vi "AK Befehl Auswerten_MEXA.vi"(10 "Array":string[](array[string])) -> (2 "String für schreiben":string)   [LabVIEW 2020, in "AK-Schnittstelle.lvlib"]
uses:
  AK-Schnittstelle.lvlib
  Aktionen Stoernummern pruefen.ctl
  Aktionen Zustandsfehlerinformation.ctl
  AK Namen Aktionen.ctl
  Seiten/CalGas Aufschaltung/FGV CalGas Aktionen.ctl
  Seiten/FT-IR/Aktion FGV Rezepte wechseln.ctl
  Seiten/FT-IR/AK-manuell.ctl
  Amium PNS/Aktion FGV Amium Daten.ctl
  Seiten/System Einstellungen V2/Aktioen FGV System Konstanten.ctl
  Aktionen Gespeicherte Werte.ctl
  Seiten/System Einstellungen V2/Aktioen FGV System.ctl
  Funktionstasten/Funktionstasten-Aktion.ctl
  Funktionstasten/Zustaende.ctl
  Schedule Modul/Aktion FGV Scheduler Status.ctl
  Seiten/FT-IR/FGV FT-IR Aktionen.ctl
  Analysator Definition/FGV Analysator Definition Aktionen.ctl
  Seiten/FT-IR/FGV FT-IR Diagnose Aktionen.ctl
  Seiten/Erweiterte Konfig/Status Dichtheitstest Aktionen.ctl
  Seiten/Erweiterte Konfig/FGV PID Aktionen.ctl
  Seiten/Anlagengrenzwerte/FGV Anlagengrenzwerte Aktionen.ctl
  Funktionstasten/Betriebsart.ctl
  Amium PNS/AK Kommunikation/Amium Kommandos verwalten Aktionen.ctl
  Seiten/Log Konfig/Aktionen Trigger.ctl
  Messdaten/Aktionen FGV Messdaten.ctl
  Seiten/FT-IR/TOOLweb Interface Library/TOOLweb Rezept wechseln.vi
  Seiten/Erweiterte Konfig/Dichtheitstest.vi
  Funktionstasten/Funktionstasten.lvlib
  Seiten/Log Konfig/LogKonfig.lvlib
  Seiten/FT-IR/FT-IR.lvlib
  Seiten/FT-IR/FGV FT-IR Gasliste Aktionen.ctl
  Messdaten/Messdaten.lvlib
  Seiten/System Einstellungen V2/System Einstellungen V2.lvlib
  Seiten/Erweiterte Konfig/Erweiterte Konfig.lvlib
  Allgemein/allgemeine Sub-VIs.lvlib
  cRIO/PC/Kommunikation mit cRIO.lvlib
  Seiten/Anlagengrenzwerte/Anlagengrenzwerte.lvlib
  Seiten/FT-IR/TOOLweb Interface Library/TOOLweb Interface.lvlib
  Analysator Definition/Analysator Definition.lvlib
  Amium PNS/AK Kommunikation/AK Kommunikation.lvlib
  Seiten/CalGas Aufschaltung/CalGas Aufschaltung.lvlib
  Amium PNS/Amium PNS.lvlib
  Schedule Modul/Schedule Modul.lvlib
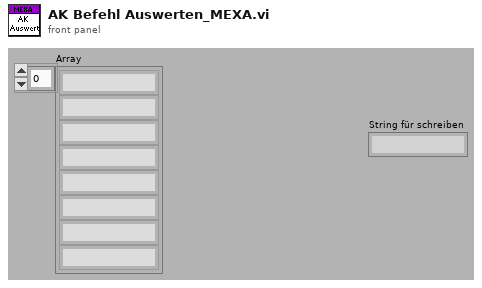
[diagram p1: front panel]
types:
  T1 = typedef "AK-Schnittstelle.lvlib/Aktionen Stoernummern pruefen.ctl" = enum16{"lesen", "prüfen"}
  T2 = typedef "AK-Schnittstelle.lvlib/Aktionen Zustandsfehlerinformation.ctl" = enum16{"OK", "Offline", "Busy", "Syntax Error", "Datenfehler"}
  T3 = typedef "AK-Schnittstelle.lvlib/AK Namen Aktionen.ctl" = enum16{"lesen", "laden", "speichern Namen", "AK Namen", "Liste erstellen", "EKFG erstellen", "speichern EKFG", "EKFG schreiben", "Neuen Eintrag erzeugen"}
  T4 = typedef "CalGas Aufschaltung.lvlib/FGV CalGas Aktionen.ctl" = enum16{"lesen", "Analysator Auswahl", "Def.CalGas", "Aufschaltung CalGas", "laden", "speichern", "KAL extrahieren"}
  T5 = typedef "FT-IR.lvlib/AK-manuell.ctl" = enum16{"manuell", "Diesel", "CNG", "Gasoline"}
  T6 = typedef "FT-IR.lvlib/Aktion FGV Rezepte wechseln.ctl" = enum16{"lesen", "Rezepte", "Rezeptindex", "Diesel", "Gasoline", "NCG", "laden", "speichern", "AK/Man"}
  T7 = typedef "Amium PNS.lvlib/Aktion FGV Amium Daten.ctl" = enum16{"lesen", "Komm Daten", "Daten", "Error", "Regler", "Grenzwerte", "laden", "speichern"}
  T8 = typedef "System Einstellungen V2.lvlib/Aktioen FGV System Konstanten.ctl" = enum16{"lesen", "laden", "speichern", "Sprache"}
  T9 = typedef "System Einstellungen V2.lvlib/Aktioen FGV System.ctl" = enum16{"lesen", "laden", "speichern", "Optionen schreiben", "Zeitstempel", "Reset BMP", "Reset SQP", "Wartung", "Werkseinstellung"}
  T10 = typedef "AK-Schnittstelle.lvlib/Aktionen Gespeicherte Werte.ctl" = enum16{"lesen", "laden", "speichern", "Seriell", "TCP", "Diverse", "AKTIV", "AK-Namen"}
  T11 = typedef "Messdaten.lvlib/Aktionen FGV Messdaten.ctl" = enum16{"lesen", "schreiben", "löschen", "Mittelwerte", "Komponente"}
  T12 = typedef "Funktionstasten.lvlib/Zustaende.ctl" = enum16{"Standby", "Pause", "Eco", "Messen", "Kalibrieren", "Spülen Filter", "Spülen Leitung", "Umgebungsluft", "0-Gas", "Cal-Gas", "CG zu PNS", "-------------", "Init 1", "Init 2", "Init 3", "Init 4", "Messen vorbereiten", "Messen durchführen", "Exit"}
  T13 = typedef "Funktionstasten.lvlib/Funktionstasten-Aktion.ctl" = enum16{"Initialisieren", "Zustand setzen", "Taste gedrückt", "Fehler speichern", "Lesen", "Manuell", "Remote", "Bitparallel", "Samplepoint", "Zeit Prüfen", "reset Umschalten"}
  T14 = typedef "Schedule Modul.lvlib/Aktion FGV Scheduler Status.ctl" = enum16{"lesen", "init", "aktiv", "inaktiv"}
  T15 = typedef "FT-IR.lvlib/FGV FT-IR Aktionen.ctl" = enum16{"lesen", "NOG setzen", "NOS setzen", "Initialisieren", "speichern", "ALLES setzen", "FT-IR Spektrum loggen", "Komm Stoppen", "Spektrum LogKonfig"}
  T16 = typedef "FT-IR.lvlib/FGV FT-IR Gasliste Aktionen.ctl" = enum16{"lesen", "Gasliste FT-IR", "Gasliste ausgelesen", "laden", "speichern", "löschen"}
  T17 = typedef "Analysator Definition.lvlib/FGV Analysator Definition Aktionen.ctl" = enum16{"lesen", "MB setzen", "MB KAL setzen", "laden"}
  T18 = typedef "FT-IR.lvlib/FGV FT-IR Diagnose Aktionen.ctl" = enum16{"Lesen", "Diagnose Schreiben", "Min Schreiben", "Max Schreiben"}
  T19 = typedef "Erweiterte Konfig.lvlib/Status Dichtheitstest Aktionen.ctl" = enum16{"lesen", "Zeitstempel", "Daten", "läuft", "Protokolldaten"}
  T20 = typedef "Erweiterte Konfig.lvlib/FGV PID Aktionen.ctl" = enum16{"Lesen", "Schreiben PID", "Schreiben Sonstige", "Dichtheitstest", "Aktionen Dicht.", "Parameter Sensor"}
  T21 = typedef "Anlagengrenzwerte.lvlib/FGV Anlagengrenzwerte Aktionen.ctl" = enum16{"Lesen", "Grenzwerte schreiben"}
  T22 = typedef "Funktionstasten.lvlib/Betriebsart.ctl" = enum16{"Manuell", "Remote", "Bitparallel"}
  T23 = typedef "Amium PNS.lvlib/AK Kommunikation.lvlib/Amium Kommandos verwalten Aktionen.ctl" = enum16{"lesen", "setzen Ende", "setzen Pos1", "senden", "initalisieren", "prüfen", "Kommandos"}
  T24 = typedef "LogKonfig.lvlib/Aktionen Trigger.ctl" = enum16{"lesen", "ALLE schreiben", "Trigger prüfen", "Trigger rücksetzen"}
  T25 = typedef "CalGas Aufschaltung.lvlib/Definition CalGas Anzeige.ctl" = cluster{"Namen":T26, "Werte":T28, "Werte 2":T28, "Einheit":T30, "Messbereiche":T32}
  T26 = typedef "CalGas Aufschaltung.lvlib/CalGas-Namen.ctl" = cluster{"Name":T27, "Name 2":T27, "Name 3":T27, "Name 4":T27, "Name 5":T27, "Name 6":T27, "Name 7":T27, "Name 8":T27, "Name 9":T27, "Name 10":T27, "Name 11":T27, "Name 12":T27}
  T27 = typedef "String - Eingabefeld.ctl" = string
  T28 = typedef "CalGas Aufschaltung.lvlib/CalGas-Werte.ctl" = cluster{"Konzentration 1":T29, "Konzentration 2":T29, "Konzentration 3":T29, "Konzentration 4":T29, "Konzentration 5":T29, "Konzentration 6":T29, "Konzentration 7":T29, "Konzentration 8":T29, "Konzentration 9":T29, "Konzentration 10":T29, "Konzentration 11":T29, "Konzentration 12":T29}
  T29 = typedef "Zahlen-Eingabefeld.ctl" = sgl
  T30 = typedef "CalGas Aufschaltung.lvlib/CalGas-Einheit.ctl" = cluster{"Einheit 1":T31, "Einheit 2":T31, "Einheit 3":T31, "Einheit 4":T31, "Einheit 5":T31, "Einheit 6":T31, "Einheit 7":T31, "Einheit 8":T31, "Einheit 9":T31, "Einheit 10":T31, "Einheit 11":T31, "Einheit 12":T31}
  T31 = typedef "Auswahlfeld.ctl" = u16
  T32 = typedef "CalGas Aufschaltung.lvlib/CalGas-Messbereiche.ctl" = cluster{"Messbereich 1":T31, "Messbereich 2":T31, "Messbereich 3":T31, "Messbereich 4":T31, "Messbereich 5":T31, "Messbereich 6":T31, "Messbereich 7":T31, "Messbereich 8":T31, "Messbereich 9":T31, "Messbereich 10":T31, "Messbereich 11":T31, "Messbereich 12":T31}
  T33 = typedef "Amium PNS.lvlib/Daten Cluster.ctl" = cluster{"Amium Zustände":T34, "Samplepoint am PNS":i16, "Gerätekennung":string, "aktiver Samplepoint":i16[], "Messgasdruck":sgl}
  T34 = typedef "Amium PNS.lvlib/Amium Zustand.ctl" = u16
  T35 = cluster{"Modell":string, "ProjektNummer":string, "Software Version":string, "Seriennummer":string}
  T36 = typedef "System Einstellungen V2.lvlib/Optionen.ctl" = cluster{"Störmeldep.":bool, "Betriebszustände":bool, "AK in ppm":bool, "log Cal-Gas":bool, "log 0-Gas":bool, "Durchflusssensor 0-5V":bool, "PNS?":bool, "Mit N2 spülen":bool, "TRE08":bool, "Amium 10-Fach":bool, "Verticale Scrollbar aktiv":bool, "Loggingtakt":bool, "AK Rezeptwechsel gleich wie MKS":bool, "NG ECO":bool}
  T37 = typedef "AK-Schnittstelle.lvlib/Diverse gespeicherte Werte.ctl" = cluster{"Kalibriergaseingang":i16, "SamplePoint":i16, "CalGas zu PNS":i16, "Gas-Reihenfolge":i16[], "Zeit 0-Gas":sgl, "Zeit CalGas":sgl, "AK Befehlssatz":T38}
  T38 = typedef "AK-Schnittstelle.lvlib/AK Befehlssatz.ctl" = enum16{"MEXA", "IAG v1.4", "AVL (Puma)", "PEUS"}
  T39 = typedef "String - Ausgabefeld.ctl" = string
  T40 = typedef "Analysator Definition.lvlib/Betriebsdaten Komponente.ctl" = cluster{"Namen":string[], "MB Namen":string[], "Einheit":string, "MB Aktuell":u16, "MB Endwert":u16, "CalGase":u16[], "MB für KAL":u16[], "CG für KAL":u16[]}
  T41 = typedef "Verwaltung - cRIO.lvlib/TC Eingaenge.ctl" = cluster{"TC0: Reserve":sgl, "TC1: HL zu FT-IR":sgl, "TC2: HL Extern SP1":sgl, "TC3: HL Extern SP2":sgl, "TC4: Reserve":sgl, "TC5: Reserve":sgl, "TC6: Reserve":sgl, "TC7: Reserve":sgl, "TC8: FT-IR":sgl, "TC9: Reserve":sgl, "TC10: Schaltschrank":sgl, "TC11: Umgebung":sgl}
  T42 = typedef "Verwaltung - cRIO.lvlib/Analog Eingaenge.ctl" = cluster{"AI0: Durchfluss FT-IR":sgl, "AI1: Druck Ausgang":sgl, "AI2: Umgebungsdruck":sgl, "AI3: Druck FT-IR":sgl, "AI4: Druck CalGas":sgl, "AI5: Reserve":sgl, "AI6: Reserve":sgl, "AI7: Reserve":sgl, "Rohwert Durchfluss FT-IR":sgl, "Rohwert Druck Ausgang":sgl, "Rohwert Umgebungsdruck":sgl, "Rohwert Druck FT-IR":sgl, "Rohwert Druck CalGas":sgl, "Rohwert AI5":sgl, "Rohwert AI6":sgl, "Rohwert AI7":sgl, "Rohwert Diffdruck mbar FTIR":sgl}
  T43 = typedef "Erweiterte Konfig.lvlib/Sonstige Parameter.ctl" = cluster{"Lüfter langsam":sgl, "Lüfter schnell":sgl, "FT-IR Kühlung Soll":sgl, "FT-IR Kühlung Max":sgl, "Überwachung":T31, "Befüllung aktiv":T44, "Stickstoff Befüllzeit":sgl, "Befüllintervall":sgl, "Kalibrierwert FT-IR":sgl, "Offset Ausgang":sgl, "Offset FT-IR":sgl, "Offset Druck FT-IR":sgl, "Dichtheitstest Zeit":sgl, "Dichtheitstest Abfall":sgl, "Dichtheitstest Umfang":T45, "Offset Umgebung":sgl, "Max Taupunkt":sgl, "Pumpendrehzahl":sgl, "ext. Befüllung":T44, "Ext. Stickstoff Befüllzeit":sgl}
  T44 = typedef "LogKonfig.lvlib/Auswahlfeld aktiviert-deaktiviert.ctl" = u16
  T45 = typedef "Erweiterte Konfig.lvlib/Dichtheitstest Umfang.ctl" = u16
  T46 = typedef "Anlagengrenzwerte.lvlib/Anlagen-Grenzwerte Anzeige.ctl" = cluster{"Eingangsdruck FT-IR:":T47, "Durchfluss FT-IR:":T47, "Durchfluss CalGas:":T47, "Druck Ausgang:":T47, "Druck Kalter Block:":T47, "Heizleitungen intern:":T47, "Heizleitung zu FT-IR:":T47, "Heizung Filterblock:":T47, "Heizung Pumpe:":T47, "Heizleitung Extern SP1:":T47, "Heizleitung Extern SP2:":T47, "FT-IR Heizung Messzelle:":T47, "Schaltschranktemperatur:":T47, "Gaskühler:":T47}
  T47 = typedef "Anlagengrenzwerte.lvlib/Anlagen-Parameter Anzeige.ctl" = cluster{"Sollwert":sgl, "Warn-Min":sgl, "Warn-Max":sgl, "Abschalt-Min":sgl, "Abschalt-Max":sgl, "Regler":u16}
  T48 = typedef "LogKonfig.lvlib/Element Triggerereignisse.ctl" = cluster{"Trigger verwenden":T44, "Messwert":u16, "kl./gr.":u16, "Wert":sgl, "Puffergröße":sgl}
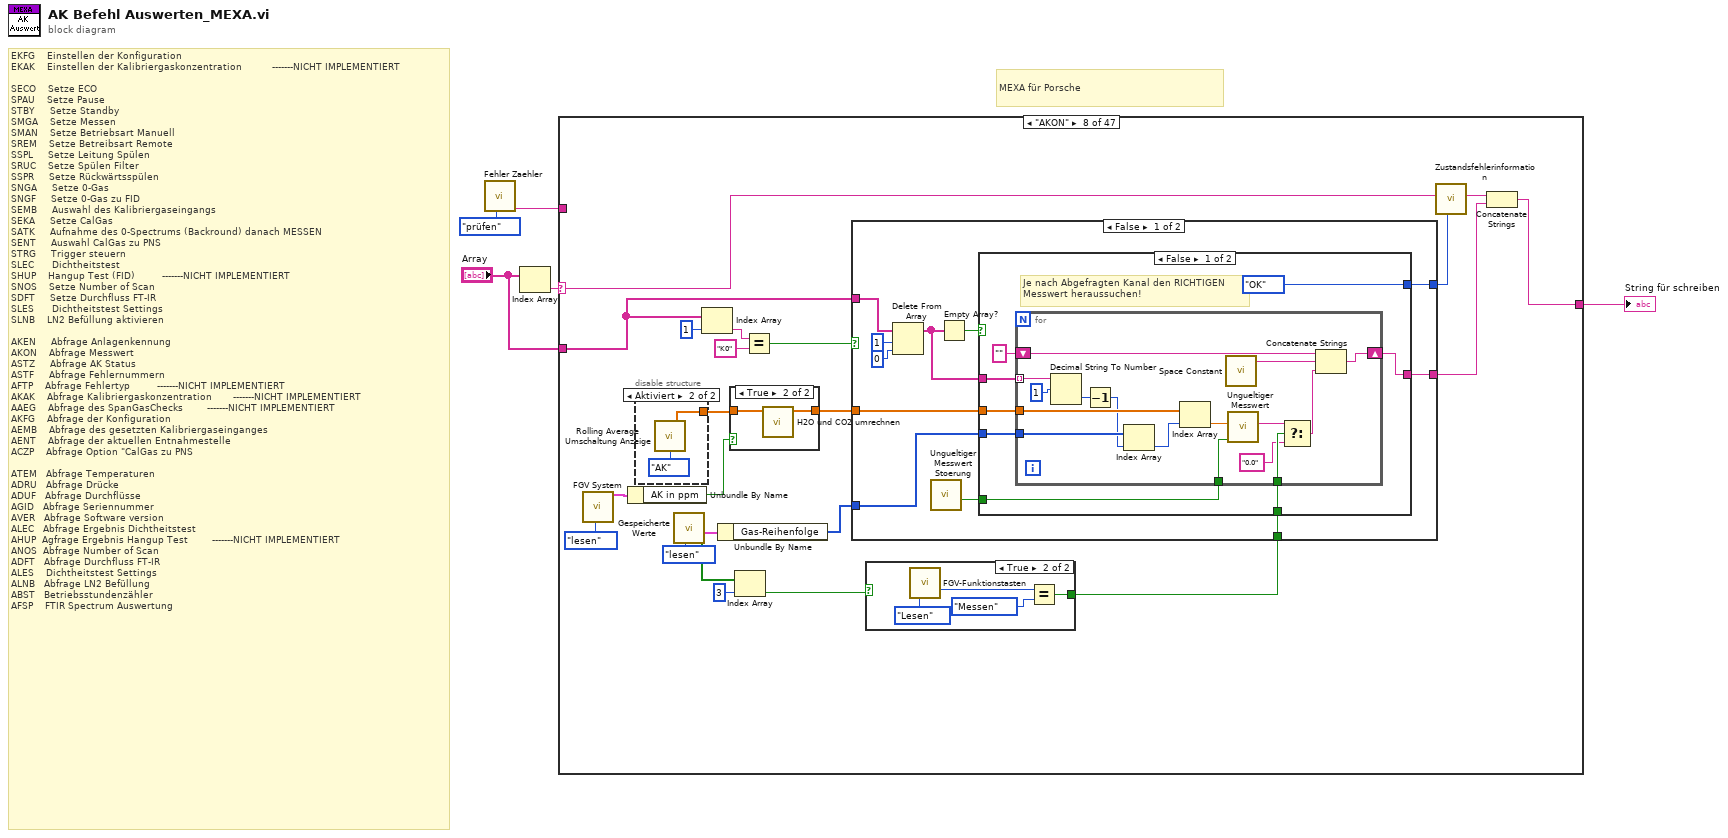
[diagram p0: block diagram]
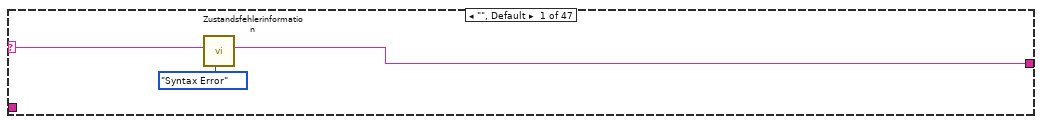
[diagram p2: hidden frame]
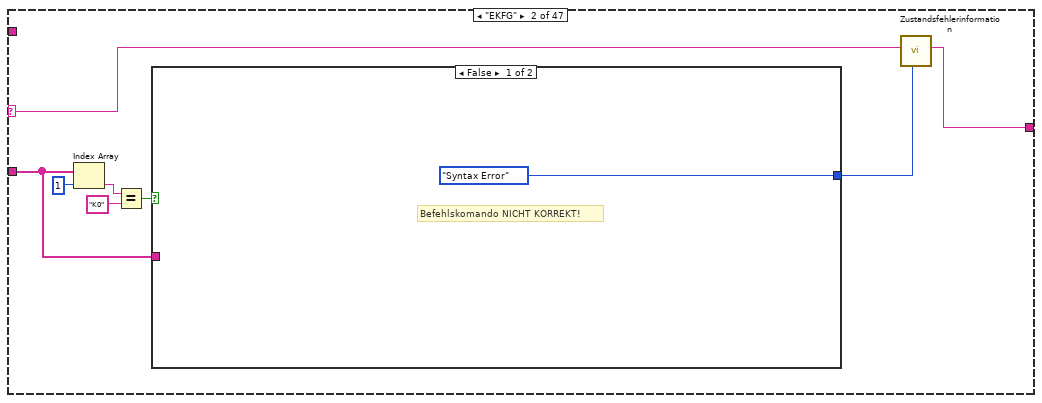
[diagram p3: hidden frame]
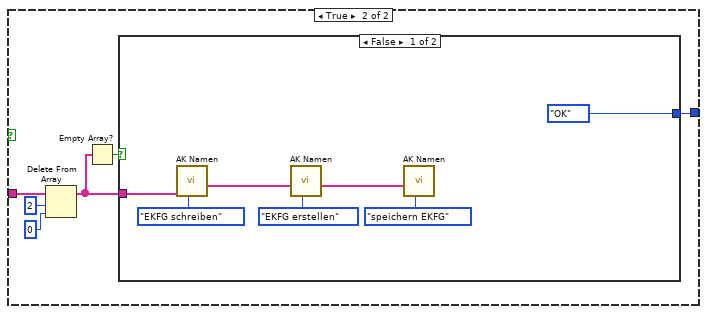
[diagram p4: hidden frame]
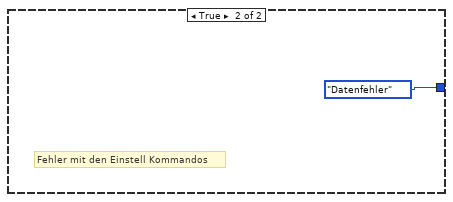
[diagram p5: hidden frame]
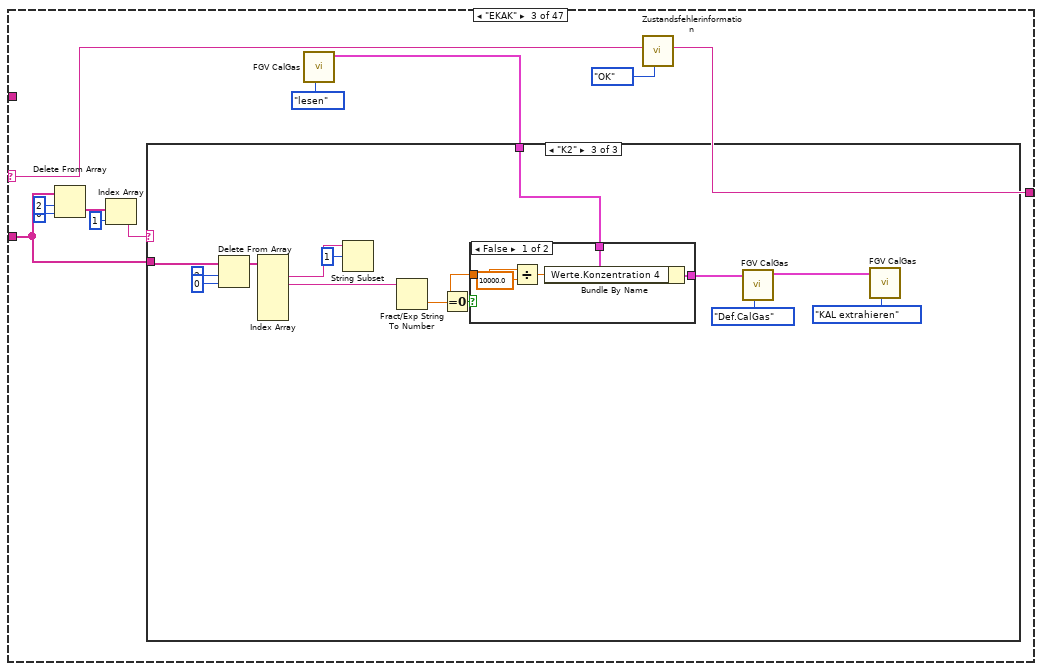
[diagram p6: hidden frame]
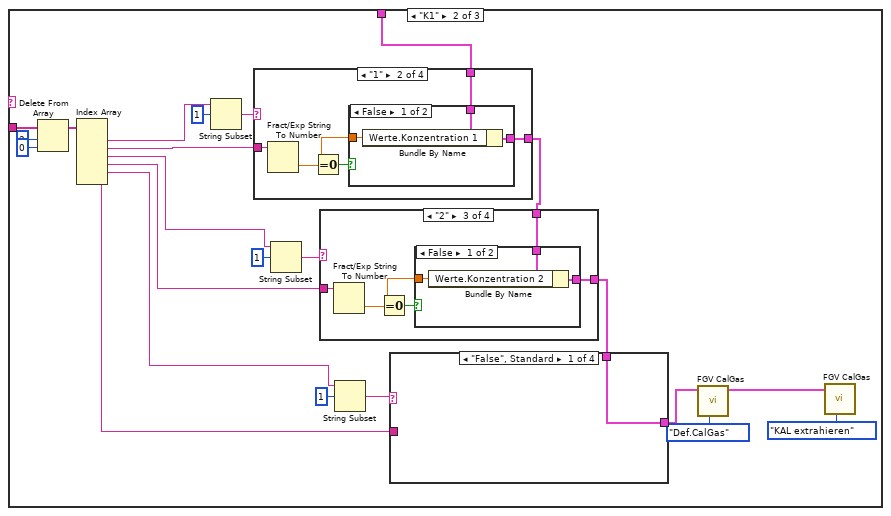
[diagram p8: hidden frame]
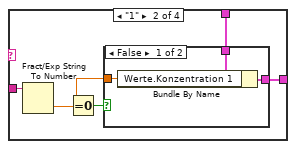
[diagram p9: hidden frame]
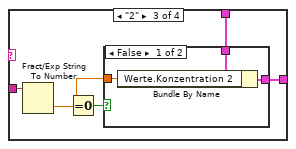
[diagram p11: hidden frame]
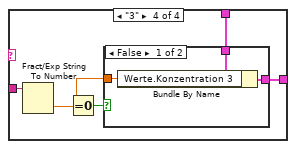
[diagram p13: hidden frame]
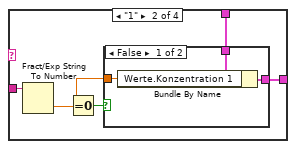
[diagram p16: hidden frame]
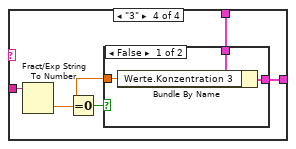
[diagram p19: hidden frame]
diagram:
  # "MEXA für Porsche"
  # "EKFG    Einstellen der Konfiguration\nEKAK    Einstellen der Kalibriergaskonzentration          -------NICHT IMPLEMENTIERT\n\nSECO    Setze ECO\nSPAU    Setze Pause\nSTBY     Setze Standby\nSMGA    Setze Messen\nSMAN    Setze Betriebsart Manuell\nSREM    Setze Betreibsart Remote\nSSPL     Setze Leitung Spülen\nSRUC    Setze Spülen Filter\nSSPR     Setze Rückwärtsspülen\nSNGA     Setze 0-Gas\nSNGF     Setze 0-Gas zu FID\nSEMB     Auswahl des Kalibriergaseingangs\nSEKA     Setze CalGas\nSATK     Aufnahme des 0-Spectrums (Backround) danach MESSEN\nSENT     Auswahl CalGas zu PNS\nSTRG     Trigger steuern\nSLEC      Dichtheitstest\nSHUP    Hangup Test (FID)         -------NICHT IMPLEMENTIERT\nSNOS    Setze Number of Scan\nSDFT     Setze Durchfluss FT-IR\nSLES      Dichtheitstest Settings\nSLNB    LN2 Befüllung aktivieren\n\nAKEN     Abfrage Anlagenkennung\nAKON    Abfrage Messwert\nASTZ     Abfrage AK Status\nASTF     Abfrage Fehlernummern\nAFTP    Abfrage Fehlertyp         -------NICHT IMPLEMENTIERT\nAKAK    Abfrage Kalibriergaskonzentration       -------NICHT IMPLEMENTIERT\nAAEG    Abfrage des SpanGasChecks        -------NICHT IMPLEMENTIERT\nAKFG    Abfrage der Konfiguration\nAEMB    Abfrage des gesetzten Kalibriergaseinganges\nAENT    Abfrage der aktuellen Entnahmestelle\nACZP    Abfrage Option \"CalGas zu PNS\n\nATEM   Abfrage Temperaturen\nADRU   Abfrage Drücke\nADUF   Abfrage Durchflüsse\nAGID   Abfrage Seriennummer\nAVER   Abfrage Software version\nALEC   Abfrage Ergebnis Dichtheitstest\nAHUP  Agfrage Ergebnis Hangup Test        -------NICHT IMPLEMENTIERT\nANOS  Abfrage Number of Scan\nADFT   Abfrage Durchfluss FT-IR\nALES    Dichtheitstest Settings\nALNB   Abfrage LN2 Befüllung\nABST   Betriebsstundenzähler\nAFSP    FTIR Spectrum Auswertung"
  n1 = call "Fehler Zaehler.vi"("Aktionen"=Aktionen_Stoernummern_pruefen."prüfen") -> ("Fehlerzähler"=w3:string)  [unwired: 7 in, 3 out]
  n2 = Index Array(array="Array") -> (element=w2:string)  [unwired: 1 in]
  n3 = case shown="\"AKON\"" w2 {
    selector: w2 -> [w7 w15 w39 w180 w211 w249 w262 w285 w360 w383 w390 w399 w411 w442 w451 w469 w483 w506 w520 w527 w535 w550 w571 w582 w591 w601 w615 w623 w626 w629 w632 w642 w652 w656 w666 w670 w672 w685 w691 w710 w727 w732 w754 w793 w817 w868 w899]
    tunnel: [w6 w14 w38 w171 w210 w242 w264 w286 w362 w385 w392 w401 w413 w444 w453 w459 w479 w501 w517 w522 w531 w543 w569 w584 w593 w603 w613 w622 w625 w628 w631 w641 w651 w655 w665 w669 w671 w684 w690 w709 w726 w731 w753 w792 w816 w867 w898] -> w5
    tunnel: w3 -> [_ _ _ _ _ _ _ _ _ _ _ _ _ _ _ _ _ _ _ _ _ _ _ _ _ _ _ _ _ _ _ _ _ _ _ _ _ _ _ _ _ _ _ _ _ _ _]
    tunnel: "Array" -> [_ w16 w32 w181 w212 _ _ w276 _ _ _ _ _ _ _ _ _ _ _ _ _ _ _ _ _ _ _ _ _ _ _ w634 w644 _ w664 _ _ _ w689 _ _ w730 w752 _ w815 w866 w897]
    frame "", Default {
      n4 = call "Zustandsfehlerinformation.vi"("Aktionen"=Aktionen_Zustandsfehlerinformation."Syntax Error", "String"=w7) -> ("String"=w6:string)  [unwired: 9 in]
    }
    frame "EKFG" {
      n5 = Index Array(array=w16, index=1 ("Index")) -> (element=w12:string)
      n6 = Equal?(x=w12, y="K0") -> (x = y?=w10:bool)
      n7 = case shown="False" w10 {
        tunnel: w16 -> [_ w21]
        tunnel: [Aktionen_Zustandsfehlerinformation."Syntax Error" ("Aktionen") w18] -> w9
        frame False {
          # "Befehlskomando NICHT KORREKT!"
        }
        frame True {
          n8 = Delete From Array(array=w21, length=2 ("Länge"), index=0 ("Index")) -> (array with subset deleted=w20:string[])  [unwired: 1 out]
          n9 = Empty Array?(array=w20) -> (empty?=w19:bool)
          n10 = case shown="False" w19 {
            tunnel: w20 -> [w29 _]
            tunnel: [Aktionen_Zustandsfehlerinformation."OK" ("Aktionen") Aktionen_Zustandsfehlerinformation."Datenfehler" ("Aktionen")] -> w18
            frame False {
              n11 = call "AK Namen.vi"("Aktionen"=AK_Namen_Aktionen."EKFG schreiben", "EKFG Liste"=w29) -> ("AK Namen"=w26:string[])  [unwired: 6 in, 3 out]
              n12 = call "AK Namen.vi"("Aktionen"=AK_Namen_Aktionen."EKFG erstellen", "AK Namen"=w26) -> ("AK Namen"=w24:string[])  [unwired: 6 in, 3 out]
              n13 = call "AK Namen.vi"("Aktionen"=AK_Namen_Aktionen."speichern EKFG", "AK Namen"=w24) -> ()  [unwired: 6 in, 4 out]
            }
            frame True {
              # "Fehler mit den Einstell Kommandos"
            }
          }
        }
      }
      n14 = call "Zustandsfehlerinformation.vi"("Aktionen"=w9, "String"=w15) -> ("String"=w14:string)  [unwired: 9 in]
    }
    frame "EKAK" {
      n15 = Delete From Array(array=w32, length=2 ("Länge"), index=0 ("Index")) -> (deleted portion=w35:string[])  [unwired: 1 out]
      n16 = Index Array(array=w35, index=1 ("Index")) -> (element=w34:string)
      n17 = call "FGV CalGas.vi"("Aktionen"=FGV_CalGas_Aktionen."lesen") -> ("Def.CalGas"=w41:T25)  [unwired: 6 in, 4 out]
      n18 = case shown="\"K2\"" w34 {
        tunnel: w41 -> [_ w65 w163]
        tunnel: w32 -> [_ w51 w156]
        frame "False", Default {
        }
        frame "K1" {
          n19 = Delete From Array(array=w51, length=2 ("Länge"), index=0 ("Index")) -> (array with subset deleted=w52:string[])  [unwired: 1 out]
          n20 = Index Array(array=w52) -> (element #1=w62:string, element #2=w61:string, element #3=w45:string, element #4=w57:string, element #5=w43:string, element #6=w54:string)  [unwired: 6 in]
          n21 = String Subset(string=w62, offset (0)=1 ("Offset (0)")) -> (substring=w63:string)  [unwired: 1 in]
          n22 = case shown="\"1\"" w63 {
            tunnel: w65 -> [w122 w127 w136 w145]
            tunnel: w61 -> [_ w126 w135 w144]
            tunnel: [w122 w125 w134 w143] -> w56
            frame "False", Default {
            }
            frame "1" {
              n23 = Fract/Exp String To Number(string=w126) -> (number=w124:dbl)  [unwired: 3 in, 1 out]
              n24 = Equal To 0?(x=w124) -> (x = 0?=w123:bool)
              n25 = case shown="False" w123 {
                tunnel: w127 -> [w130 w131]
                tunnel: [w129 w131] -> w125
                tunnel: w124 -> [w128 _]
                frame False {
                  n26 = Bundle By Name(cluster=w130, "Werte.Konzentration 1"=w128) -> (w129:T25)
                }
                frame True {
                }
              }
            }
            frame "2" {
              n27 = Fract/Exp String To Number(string=w135) -> (number=w133:dbl)  [unwired: 3 in, 1 out]
              n28 = Equal To 0?(x=w133) -> (x = 0?=w132:bool)
              n29 = case shown="False" w132 {
                tunnel: w136 -> [w139 w140]
                tunnel: [w138 w140] -> w134
                tunnel: w133 -> [w137 _]
                frame False {
                  n30 = Bundle By Name(cluster=w139, "Werte.Konzentration 2"=w137) -> (w138:T25)
                }
                frame True {
                }
              }
            }
            frame "3" {
              n31 = Fract/Exp String To Number(string=w144) -> (number=w142:dbl)  [unwired: 3 in, 1 out]
              n32 = Equal To 0?(x=w142) -> (x = 0?=w141:bool)
              n33 = case shown="False" w141 {
                tunnel: w145 -> [w148 w149]
                tunnel: [w147 w149] -> w143
                tunnel: w142 -> [w146 _]
                frame False {
                  n34 = Bundle By Name(cluster=w148, "Werte.Konzentration 3"=w146) -> (w147:T25)
                }
                frame True {
                }
              }
            }
          }
          n35 = String Subset(string=w45, offset (0)=1 ("Offset (0)")) -> (substring=w46:string)  [unwired: 1 in]
          n36 = case shown="\"2\"" w46 {
            tunnel: w56 -> [w94 w99 w108 w117]
            tunnel: w57 -> [_ w98 w107 w116]
            tunnel: [w94 w97 w104 w115] -> w55
            frame "False", Default {
            }
            frame "1" {
              n37 = Fract/Exp String To Number(string=w98) -> (number=w96:dbl)  [unwired: 3 in, 1 out]
              n38 = Equal To 0?(x=w96) -> (x = 0?=w95:bool)
              n39 = case shown="False" w95 {
                tunnel: w99 -> [w102 w103]
                tunnel: [w101 w103] -> w97
                tunnel: w96 -> [w100 _]
                frame False {
                  n40 = Bundle By Name(cluster=w102, "Werte.Konzentration 1"=w100) -> (w101:T25)
                }
                frame True {
                }
              }
            }
            frame "2" {
              n41 = Fract/Exp String To Number(string=w107) -> (number=w106:dbl)  [unwired: 3 in, 1 out]
              n42 = Equal To 0?(x=w106) -> (x = 0?=w105:bool)
              n43 = case shown="False" w105 {
                tunnel: w108 -> [w111 w112]
                tunnel: [w110 w112] -> w104
                tunnel: w106 -> [w109 _]
                frame False {
                  n44 = Bundle By Name(cluster=w111, "Werte.Konzentration 2"=w109) -> (w110:T25)
                }
                frame True {
                }
              }
            }
            frame "3" {
              n45 = Fract/Exp String To Number(string=w116) -> (number=w114:dbl)  [unwired: 3 in, 1 out]
              n46 = Equal To 0?(x=w114) -> (x = 0?=w113:bool)
              n47 = case shown="False" w113 {
                tunnel: w117 -> [w120 w121]
                tunnel: [w119 w121] -> w115
                tunnel: w114 -> [w118 _]
                frame False {
                  n48 = Bundle By Name(cluster=w120, "Werte.Konzentration 3"=w118) -> (w119:T25)
                }
                frame True {
                }
              }
            }
          }
          n49 = String Subset(string=w43, offset (0)=1 ("Offset (0)")) -> (substring=w44:string)  [unwired: 1 in]
          n50 = case shown="\"False\", Standard" w44 {
            tunnel: w55 -> [w66 w71 w80 w89]
            tunnel: w54 -> [_ w70 w79 w88]
            tunnel: [w66 w69 w78 w87] -> w53
            frame "False", Default {
            }
            frame "1" {
              n51 = Fract/Exp String To Number(string=w70) -> (number=w68:dbl)  [unwired: 3 in, 1 out]
              n52 = Equal To 0?(x=w68) -> (x = 0?=w67:bool)
              n53 = case shown="False" w67 {
                tunnel: w71 -> [w74 w75]
                tunnel: [w73 w75] -> w69
                tunnel: w68 -> [w72 _]
                frame False {
                  n54 = Bundle By Name(cluster=w74, "Werte.Konzentration 1"=w72) -> (w73:T25)
                }
                frame True {
                }
              }
            }
            frame "2" {
              n55 = Fract/Exp String To Number(string=w79) -> (number=w77:dbl)  [unwired: 3 in, 1 out]
              n56 = Equal To 0?(x=w77) -> (x = 0?=w76:bool)
              n57 = case shown="False" w76 {
                tunnel: w80 -> [w83 w84]
                tunnel: [w82 w84] -> w78
                tunnel: w77 -> [w81 _]
                frame False {
                  n58 = Bundle By Name(cluster=w83, "Werte.Konzentration 2"=w81) -> (w82:T25)
                }
                frame True {
                }
              }
            }
            frame "3" {
              n59 = Fract/Exp String To Number(string=w88) -> (number=w86:dbl)  [unwired: 3 in, 1 out]
              n60 = Equal To 0?(x=w86) -> (x = 0?=w85:bool)
              n61 = case shown="False" w85 {
                tunnel: w89 -> [w92 w93]
                tunnel: [w91 w93] -> w87
                tunnel: w86 -> [w90 _]
                frame False {
                  n62 = Bundle By Name(cluster=w92, "Werte.Konzentration 3"=w90) -> (w91:T25)
                }
                frame True {
                }
              }
            }
          }
          n63 = call "FGV CalGas.vi"("Aktionen"=FGV_CalGas_Aktionen."Def.CalGas", "Def.CalGas neu"=w53) -> ("Def.CalGas"=w60:T25)  [unwired: 5 in, 4 out]
          n64 = call "FGV CalGas.vi"("Aktionen"=FGV_CalGas_Aktionen."KAL extrahieren", "Def.CalGas neu"=w60) -> ()  [unwired: 5 in, 5 out]
        }
        frame "K2" {
          n65 = Delete From Array(array=w156, length=2 ("Länge"), index=0 ("Index")) -> (array with subset deleted=w159:string[])  [unwired: 1 out]
          n66 = Index Array(array=w159) -> (element #1=w155:string, element #2=w154:string)  [unwired: 6 in, 4 out]
          n67 = String Subset(string=w155, offset (0)=1 ("Offset (0)")) -> ()  [unwired: 1 in, 1 out]
          n68 = Fract/Exp String To Number(string=w154) -> (number=w161:dbl)  [unwired: 3 in, 1 out]
          n69 = Equal To 0?(x=w161) -> (x = 0?=w160:bool)
          n70 = case shown="False" w160 {
            tunnel: w163 -> [w168 w169]
            tunnel: [w167 w169] -> w150
            tunnel: w161 -> [w166 _]
            frame False {
              n71 = Divide(x=w166, y=10000.0) -> (x/y=w165:dbl)
              n72 = Bundle By Name(cluster=w168, "Werte.Konzentration 4"=w165) -> (w167:T25)
            }
            frame True {
            }
          }
          n73 = call "FGV CalGas.vi"("Aktionen"=FGV_CalGas_Aktionen."Def.CalGas", "Def.CalGas neu"=w150) -> ("Def.CalGas"=w153:T25)  [unwired: 5 in, 4 out]
          n74 = call "FGV CalGas.vi"("Aktionen"=FGV_CalGas_Aktionen."KAL extrahieren", "Def.CalGas neu"=w153) -> ()  [unwired: 5 in, 5 out]
        }
      }
      n75 = call "Zustandsfehlerinformation.vi"("Aktionen"=Aktionen_Zustandsfehlerinformation."OK", "String"=w39) -> ("String"=w38:string)  [unwired: 9 in]
    }
    frame "AKAK" {
      n76 = Index Array(array=w181, index #1=1 ("Index")) -> (element #1=w176:string, element #2=w175:string, element #3=w174:string)  [unwired: 2 in]
      n77 = call "FGV CalGas.vi"("Aktionen"=FGV_CalGas_Aktionen."lesen") -> ("Def.CalGas"=w173:T25)  [unwired: 6 in, 4 out]
      n78 = case shown="\"K1\"" w176 {
        tunnel: w175 -> [_ _ _]
        tunnel: w174 -> [_ _ _]
        tunnel: w173 -> [_ w192 w204]
        tunnel: [_ w183 w199] -> w170
        frame "False", Default {
        }
        frame "K1" {
          n79 = Unbundle By Name(w192) -> ("Werte.Konzentration 1"=w191:T29, "Werte.Konzentration 2"=w190:T29, "Werte.Konzentration 3"=w189:T29)
          n80 = Build Array("M1", "M2", "M3") -> (w184:string[])
          n81 = Build Array(w191, w190, w189) -> (w185:T29[])
          n82 = for {
            tunnel: w185 -> [w198] mode=indexing
            tunnel: w184 -> [w197] mode=indexing
            shift-right: [w195] -> w183
            shift-left: "" -> [w193]
            n83 = Number To Fractional String(number=w198) -> (F-format string=w196:string)  [unwired: 3 in]
            n84 = call <vilib>:"Space Constant.vi"() -> ("String"=w194:string)
            n85 = Concatenate Strings(w193, w194, w197, w194, w196) -> (w195:string)
          }
        }
        frame "K2" {
          n86 = Unbundle By Name(w204) -> ("Werte.Konzentration 4"=w203:T29)
          n87 = Number To Fractional String(number=w203) -> (F-format string=w201:string)  [unwired: 3 in]
          n88 = call <vilib>:"Space Constant.vi"() -> ("String"=w200:string)
          n89 = Concatenate Strings(w200, "M1", w200, w201) -> (w199:string)
        }
      }
      n90 = call "Zustandsfehlerinformation.vi"("Aktionen"=Aktionen_Zustandsfehlerinformation."OK", "String"=w180) -> ("String"=w179:string)  [unwired: 9 in]
      n91 = Concatenate Strings(w179, w170) -> (w171:string)
    }
    frame "SRCP" {
      n92 = Index Array(array=w212, index=1 ("Index")) -> (element=w208:string)
      n93 = Equal?(x=w208, y="K0") -> (x = y?=w206:bool)
      n94 = case shown="True" w206 {
        tunnel: w212 -> [_ w217]
        tunnel: [Aktionen_Zustandsfehlerinformation."Syntax Error" ("Aktionen") w214] -> w205
        frame False {
          # "Befehlskomando NICHT KORREKT!"
        }
        frame True {
          n95 = Delete From Array(array=w217, length=2 ("Länge"), index=0 ("Index")) -> (array with subset deleted=w216:string[])  [unwired: 1 out]
          n96 = Empty Array?(array=w216) -> (empty?=w215:bool)
          n97 = case shown="False" w215 {
            tunnel: w216 -> [w221 _]
            tunnel: [w222 Aktionen_Zustandsfehlerinformation."Datenfehler" ("Aktionen")] -> w214
            frame False {
              n98 = Index Array(array=w221) -> (element=w220:string)  [unwired: 1 in]
              n99 = case shown="\"0\", Standard" w220 {
                tunnel: [Aktionen_Zustandsfehlerinformation."OK" ("Aktionen") Aktionen_Zustandsfehlerinformation."Syntax Error" ("Aktionen") Aktionen_Zustandsfehlerinformation."OK" ("Aktionen") Aktionen_Zustandsfehlerinformation."OK" ("Aktionen")] -> w222
                frame "CNG" {
                  n100 = call "FGV Rezepte wechseln.vi"("AK/man"=AK-manuell."CNG", "Aktion"=Aktion_FGV_Rezepte_wechseln."AK/Man") -> ("error out"=w225:errorcluster)  [unwired: 7 in, 6 out]
                  n101 = flat-sequence {
                    tunnel: w225 -> [_]
                    frame #0 {
                      n102 = vi-ref "FT-IR.lvlib:TOOLweb Interface.lvlib:TOOLweb Rezept wechseln.vi"() -> (w227:refnum<vi>)
                      n103 = call "VI Pop Up.vi"("VI Referenz"=w227) -> ()  [unwired: 10 in, 1 out]
                    }
                  }
                }
                frame "0", Default {
                }
                frame "DIESEL" {
                  n104 = call "FGV Rezepte wechseln.vi"("AK/man"=AK-manuell."Diesel", "Aktion"=Aktion_FGV_Rezepte_wechseln."AK/Man") -> ("error out"=w231:errorcluster)  [unwired: 7 in, 6 out]
                  n105 = flat-sequence {
                    tunnel: w231 -> [_]
                    frame #0 {
                      n106 = vi-ref "FT-IR.lvlib:TOOLweb Interface.lvlib:TOOLweb Rezept wechseln.vi"() -> (w233:refnum<vi>)
                      n107 = call "VI Pop Up.vi"("VI Referenz"=w233) -> ()  [unwired: 10 in, 1 out]
                    }
                  }
                }
                frame "GASOLINE" {
                  n108 = call "FGV Rezepte wechseln.vi"("AK/man"=AK-manuell."Gasoline", "Aktion"=Aktion_FGV_Rezepte_wechseln."AK/Man") -> ("error out"=w236:errorcluster)  [unwired: 7 in, 6 out]
                  n109 = flat-sequence {
                    tunnel: w236 -> [_]
                    frame #0 {
                      n110 = vi-ref "FT-IR.lvlib:TOOLweb Interface.lvlib:TOOLweb Rezept wechseln.vi"() -> (w238:refnum<vi>)
                      n111 = call "VI Pop Up.vi"("VI Referenz"=w238) -> ()  [unwired: 10 in, 1 out]
                    }
                  }
                }
              }
            }
            frame True {
              # "Fehler mit den Einstell Kommandos"
            }
          }
        }
      }
      n112 = call "Zustandsfehlerinformation.vi"("Aktionen"=w205, "String"=w211) -> ("String"=w210:string)  [unwired: 9 in]
    }
    frame "AENT" {
      n113 = call "FGV Amium Daten.vi"("Aktion"=Aktion_FGV_Amium_Daten."lesen") -> ("Amium Daten"=w246:T33)  [unwired: 9 in, 5 out]
      n114 = Unbundle By Name(w246) -> ("aktiver Samplepoint"=w244:i16[])
      n115 = call "Zustandsfehlerinformation.vi"("Aktionen"=Aktionen_Zustandsfehlerinformation."OK", "String"=w249) -> ("String"=w247:string)  [unwired: 9 in]
      n116 = for {
        tunnel: w244 -> [w254] mode=indexing
        shift-right: [w252] -> w243
        shift-left: "" -> [w250]
        n117 = call <vilib>:"Space Constant.vi"() -> ("String"=w251:string)
        n118 = Number To Decimal String(number=w254) -> (decimal integer string=w253:string)  [unwired: 1 in]
        n119 = Concatenate Strings(w253, w251, w250) -> (w252:string)
      }
      n120 = call <vilib>:"Space Constant.vi"() -> ("String"=w241:string)
      n121 = Concatenate Strings(w247, w241, w243) -> (w242:string)
    }
    frame "AKEN" {
      n122 = call "Zustandsfehlerinformation.vi"("Aktionen"=Aktionen_Zustandsfehlerinformation."OK", "String"=w262) -> ("String"=w261:string)  [unwired: 9 in]
      n123 = call "FGV System Konstanten.vi"("Aktionen"=Aktioen_FGV_System_Konstanten."lesen") -> ("Cluster out"=w257:T35)  [unwired: 6 in, 4 out]
      n124 = Unbundle By Name(w257) -> ("Seriennummer"=w256:string, "Software Version"=w255:string)
      n125 = call <vilib>:"Space Constant.vi"() -> ("String"=w258:string)
      n126 = Concatenate Strings(w261, w258, "IAG-Versa06" ("String"), w258, w256, w258, w255) -> (w264:string)
    }
    frame "AKON" {
      n127 = call "FGV System.vi"("Aktionen"=Aktioen_FGV_System."lesen") -> ("Optionen"=w271:T36)  [unwired: 12 in, 6 out]
      n128 = Unbundle By Name(w271) -> ("AK in ppm"=w273:bool)
      n129 = disable-structure shown="Aktiviert" {
        disable-tunnel: [w288 w290] -> w265
        frame Disabled {
          n130 = call "FGV Messdaten.vi"("Aktionen"=Aktionen_FGV_Messdaten."lesen") -> ("Aktuelle Messwerte"=w288:sgl[])  [unwired: 6 in, 8 out]
        }
        frame Enabled {
          n131 = call "Rolling Average Umschaltung Anzeige.vi"("Aktion"=enum16{"AK", "IAG Software"}."AK") -> ("Aktuelle Messwerte"=w290:sgl[])  [unwired: 9 in, 5 out]
        }
      }
      n132 = call "Gespeicherte Werte.vi"("Aktionen"=Aktionen_Gespeicherte_Werte."lesen") -> ("AKTIV?"=w268:bool[], "Diverse Werte"=w274:T37)  [unwired: 6 in, 3 out]
      n133 = Index Array(array=w276, index=1 ("Index")) -> (element=w279:string)
      n134 = Unbundle By Name(w274) -> ("Gas-Reihenfolge"=w282:i16[])
      n135 = case shown="True" w273 {
        tunnel: w265 -> [w296 w298]
        tunnel: [w296 w297] -> w270
        frame False {
        }
        frame True {
          n136 = call "H2O und CO2 umrechnen.vi"("Aktuelle Messwerte"=w298) -> ("Aktuelle Messwerte"=w297:sgl[])  [unwired: 10 in]
        }
      }
      n137 = Index Array(array=w268, index=3 ("Index")) -> (element=w266:bool)
      n138 = Equal?(x=w279, y="K0") -> (x = y?=w277:bool)
      n139 = case shown="True" w266 {
        tunnel: [TRUE w292] -> w269
        frame False {
        }
        frame True {
          n140 = call "FGV-Funktionstasten.vi"("Aktion"=Funktionstasten-Aktion."Lesen") -> ("ausgewählte Funktion"=w294:T12)  [unwired: 7 in, 7 out]
          n141 = Equal?(x=w294, y=Zustaende."Messen") -> (x = y?=w292:bool)
        }
      }
      n142 = case shown="False" w277 {
        tunnel: w282 -> [w303 w341]
        tunnel: [w301 w339] -> w281
        tunnel: w270 -> [w302 w338]
        tunnel: w276 -> [w307 _]
        tunnel: [w305 Aktionen_Zustandsfehlerinformation."OK" ("Aktionen")] -> w275
        tunnel: w269 -> [w299 _]
        frame False {
          n143 = Delete From Array(array=w307, length=1 ("Länge"), index=0 ("Index")) -> (array with subset deleted=w304:string[])  [unwired: 1 out]
          n144 = call "Ungueltiger Messwert Stoerung.vi"() -> ("Störung Messgerät"=w300:bool)  [unwired: 11 in]
          n145 = Empty Array?(array=w304) -> (empty?=w306:bool)
          n146 = case shown="False" w306 {
            tunnel: [Aktionen_Zustandsfehlerinformation."OK" ("Aktionen") Aktionen_Zustandsfehlerinformation."Datenfehler" ("Aktionen")] -> w305
            tunnel: w304 -> [w316 _]
            tunnel: w303 -> [w315 _]
            tunnel: w302 -> [w314 _]
            tunnel: [w313 ""] -> w301
            tunnel: w300 -> [w311 _]
            tunnel: w299 -> [w310 _]
            frame False {
              # "Je nach Abgefragten Kanal den RICHTIGEN\nMesswert heraussuchen!"
              n147 = for {
                tunnel: w316 -> [w333] mode=indexing
                tunnel: w315 -> [w331]
                tunnel: w314 -> [w330]
                shift-right: [w329] -> w313
                shift-left: "" -> [w328]
                tunnel: w311 -> [w322]
                tunnel: w310 -> [w320]
                n148 = Decimal String To Number(string=w333, offset=1 ("Offset (0)")) -> (number=w327:i32)  [unwired: 1 in, 1 out]
                n149 = Decrement(x=w327) -> (x-1=w326:i32)
                n150 = Index Array(array=w331, index=w326) -> (element=w324:i16)
                n151 = Index Array(array=w330, index=w324) -> (element=w323:sgl)
                n152 = call <vilib>:"Space Constant.vi"() -> ("String"=w325:string)
                n153 = call "Ungueltiger Messwert.vi"("Stöung Messgerät"=w322, "Messwert"=w323) -> ("Messwert String"=w319:string)  [unwired: 9 in]
                n154 = Select(t=w319, s=w320, f="0.0") -> (s? t:f=w321:string)
                n155 = Concatenate Strings(w328, w325, w321) -> (w329:string)
              }
            }
            frame True {
              # "Wenn der String leer ist, dann Datenfehler"
            }
          }
        }
        frame True {
          n156 = call "Ungueltiger Messwert Stoerung.vi"() -> ("Störung Messgerät"=w336:bool)  [unwired: 11 in]
          n157 = for {
            tunnel: w341 -> [w345] mode=indexing
            shift-right: [w349] -> w339
            shift-left: "" -> [w348]
            tunnel: w338 -> [w347]
            tunnel: w336 -> [w343]
            n158 = Index Array(array=w347, index=w345) -> (element=w344:sgl)
            n159 = call "Ungueltiger Messwert.vi"("Stöung Messgerät"=w343, "Messwert"=w344) -> ("Messwert String"=w342:string)  [unwired: 9 in]
            n160 = call <vilib>:"Space Constant.vi"() -> ("String"=w346:string)
            n161 = Concatenate Strings(w348, w346, w342) -> (w349:string)
          }
        }
      }
      n162 = call "Zustandsfehlerinformation.vi"("Aktionen"=w275, "String"=w285) -> ("String"=w284:string)  [unwired: 9 in]
      n163 = Concatenate Strings(w284, w281) -> (w286:string)
    }
    frame "ASTZ" {
      n164 = call "Zustandsfehlerinformation.vi"("Aktionen"=Aktionen_Zustandsfehlerinformation."OK", "String"=w360) -> ("String"=w359:string)  [unwired: 9 in]
      n165 = call "FGV Schedule Status.vi"("Aktion"=Aktion_FGV_Scheduler_Status."lesen") -> ("Scheduler Status"=w352:bool)  [unwired: 13 in, 1 out]
      n166 = call "FGV-Funktionstasten.vi"("Aktion"=Funktionstasten-Aktion."Lesen") -> ("ausgewählte Funktion"=w350:T12, "Betriebsart"=w357:T22)  [unwired: 7 in, 6 out]
      n167 = case shown="True" w352 {
        tunnel: w350 -> [w364 _]
        tunnel: [w363 "SATK" ("String")] -> w351
        frame False {
          n168 = case shown="\"Init 4\"" w364 {
            tunnel: ["STBY" ("String") "SPAU" ("String") "SECO" ("String") "SMGA" ("String") "SATK" ("String") "SEKA" ("String") "SRUC" ("String") "SSPL" ("String") "SNGA" ("String") "SCZP" ("String") _ _ _ _ _ _ _ _] -> w363
            frame "Standby", Default {
            }
            frame "Pause" {
            }
            frame "Eco" {
            }
            frame "Messen" {
            }
            frame "Kalibrieren" {
            }
            frame "Cal-Gas" {
              # "#KaliAutoMessenBug"
            }
            frame "Spülen Filter" {
            }
            frame "Spülen Leitung" {
            }
            frame "0-Gas" {
            }
            frame "CG zu PNS" {
              # "#KaliAutoMessenBug"
            }
            frame "Init 1" {
            }
            frame "Init 2" {
            }
            frame "-------------" {
            }
            frame "Init 3" {
            }
            frame "Init 4" {
            }
            frame "Messen vorbereiten" {
            }
            frame "Messen durchführen" {
            }
            frame "Exit" {
            }
          }
        }
        frame True {
        }
      }
      n169 = case shown="\"Remote\"" w357 {
        tunnel: ["SMAN" ("String") "SREM" ("String") "SBIT" ("String")] -> w356
        frame "Manuell", Default {
        }
        frame "Remote" {
        }
        frame "Bitparallel" {
        }
      }
      n170 = call <vilib>:"Space Constant.vi"() -> ("String"=w354:string)
      n171 = Concatenate Strings(w359, w354, "KV" ("String"), w354, w356, w354, w351) -> (w362:string)
    }
    frame "ARCP" {
      n172 = call "Zustandsfehlerinformation.vi"("Aktionen"=Aktionen_Zustandsfehlerinformation."OK", "String"=w383) -> ("String"=w382:string)  [unwired: 9 in]
      n173 = call "FGV FT-IR Parameter.vi"("Aktion"=FGV_FT-IR_Aktionen."lesen") -> ("Current Recipe"=w379:string)  [unwired: 11 in, 7 out]
      n174 = call <vilib>:"Space Constant.vi"() -> ("String"=w381:string)
      n175 = Concatenate Strings(w382, w381, w379) -> (w385:string)
    }
    frame "ASTF" {
      n176 = call "Zustandsfehlerinformation.vi"("Aktionen"=Aktionen_Zustandsfehlerinformation."OK", "String"=w390) -> ("String"=w389:string)  [unwired: 9 in]
      n177 = call "Fehler Zaehler.vi"("Aktionen"=Aktionen_Stoernummern_pruefen."lesen") -> ("Fehler Nummern"=w387:string)  [unwired: 7 in, 3 out]
      n178 = call <vilib>:"Space Constant.vi"() -> ("String"=w386:string)
      n179 = Concatenate Strings(w389, w386, w387) -> (w392:string)
    }
    frame "ASTA" {
      n180 = call "Zustandsfehlerinformation.vi"("Aktionen"=Aktionen_Zustandsfehlerinformation."OK", "String"=w399) -> ("String"=w398:string)  [unwired: 9 in]
      n181 = call "Fehler Zaehler.vi"("Aktionen"=Aktionen_Stoernummern_pruefen."lesen") -> ("Fehler Nummern"=w395:string)  [unwired: 7 in, 3 out]
      n182 = Empty String/Path?(string/path=w395) -> (empty?=w394:bool)
      n183 = case shown="True" w394 {
        tunnel: ["K0" _] -> w393
        frame False {
        }
        frame True {
        }
      }
      n184 = call <vilib>:"Space Constant.vi"() -> ("String"=w396:string)
      n185 = Concatenate Strings(w398, w396, w393) -> (w401:string)
    }
    frame "AKFG" {
      n186 = call "Gespeicherte Werte.vi"("Aktionen"=Aktionen_Gespeicherte_Werte."lesen") -> ("Diverse Werte"=w407:T37)  [unwired: 6 in, 4 out]
      n187 = Unbundle By Name(w407) -> ("Gas-Reihenfolge"=w409:i16[])
      n188 = disable-structure shown="Deaktiviert" {
        disable-tunnel: [w432 _] -> _
        frame Disabled {
          n189 = call "FGV Gasliste.vi"("Aktionen"=FGV_FT-IR_Gasliste_Aktionen."lesen") -> ("Aktuelle Gasliste gesamt"=w432:T39[])  [unwired: 8 in, 2 out]
        }
        frame Enabled {
        }
      }
      n190 = call "AK Namen.vi"("Aktionen"=AK_Namen_Aktionen."lesen") -> ("AK Namen"=w403:string[])  [unwired: 7 in, 3 out]
      n191 = for {
        tunnel: w409 -> [w422] mode=indexing
        shift-right: [w425] -> w406
        shift-left: "" -> [w424]
        tunnel: w403 -> [w423]
        i -> [w416]
        n192 = Index Array(array=w423, index=w422) -> (element=w420:string)
        n193 = for {
          N: 15 -> [_]
          shift-right: [w430] -> w419
          shift-left: w420 -> [w431]
          stop <- w428 stop-if-true
          n194 = call <vilib>:"Space Constant.vi"() -> ("String"=w427:string)
          n195 = Search and Replace String(input string=w431, search string=w427, replace string="_") -> (result string=w430:string, number of replacements=w429:i32)  [unwired: 5 in, 2 out]
          n196 = Less Or Equal To 0?(x=w429) -> (x <= 0?=w428:bool)
        }
        n197 = Increment(x=w416) -> (x+1=w415:i32)
        n198 = Number To Decimal String(number=w415) -> (decimal integer string=w414:string)  [unwired: 1 in]
        n199 = call <vilib>:"Space Constant.vi"() -> ("String"=w418:string)
        n200 = Concatenate Strings(w424, w418, w419, w418, "K" ("String"), w414) -> (w425:string)
      }
      n201 = call "Zustandsfehlerinformation.vi"("Aktionen"=Aktionen_Zustandsfehlerinformation."OK", "String"=w411) -> ("String"=w410:string)  [unwired: 9 in]
      n202 = Concatenate Strings(w410, w406) -> (w413:string)
    }
    frame "AEMB" {
      n203 = call "Zustandsfehlerinformation.vi"("Aktionen"=Aktionen_Zustandsfehlerinformation."OK", "String"=w442) -> ("String"=w441:string)  [unwired: 9 in]
      n204 = call "FGV Analysator Definition.vi"("Aktionen"=FGV_Analysator_Definition_Aktionen."lesen", "Komponente"=1) -> ("Betriebsdaten Komponente"=w435:T40)  [unwired: 5 in, 4 out]
      n205 = Unbundle By Name(w435) -> ("MB Aktuell"=w434:u16)
      n206 = call <vilib>:"Space Constant.vi"() -> ("String"=w438:string)
      n207 = Number To Decimal String(number=w434) -> (decimal integer string=w439:string)  [unwired: 1 in]
      n208 = Concatenate Strings(w441, w438, "M" ("String"), w439) -> (w444:string)
    }
    frame "ACZP" {
      n209 = call "Zustandsfehlerinformation.vi"("Aktionen"=Aktionen_Zustandsfehlerinformation."OK", "String"=w451) -> ("String"=w450:string)  [unwired: 9 in]
      n210 = call "Gespeicherte Werte.vi"("Aktionen"=Aktionen_Gespeicherte_Werte."lesen") -> ("Diverse Werte"=w445:T37)  [unwired: 6 in, 4 out]
      n211 = Unbundle By Name(w445) -> ("CalGas zu PNS"=w448:i16)
      n212 = call <vilib>:"Space Constant.vi"() -> ("String"=w446:string)
      n213 = Number To Decimal String(number=w448) -> (decimal integer string=w447:string)  [unwired: 1 in]
      n214 = Concatenate Strings(w450, w446, w447) -> (w453:string)
    }
    frame "ATEM" {
      n215 = call "Zustandsfehlerinformation.vi"("Aktionen"=Aktionen_Zustandsfehlerinformation."OK", "String"=w469) -> ("String"=w458:string)  [unwired: 9 in]
      n216 = call "FGV cRIO-Daten.vi"("Aktion"=enum16{"lesen", "schreiben"}."lesen") -> ("TC Eingänge"=w454:T41)  [unwired: 9 in, 9 out]
      n217 = Unbundle By Name(w454) -> ("TC0: Reserve"=w465:sgl, "TC1: HL zu FT-IR"=w464:sgl, "TC2: HL Extern SP1"=w463:sgl, "TC3: HL Extern SP2"=w462:sgl, "TC4: Reserve"=w461:sgl, "TC5: Reserve"=w457:sgl, "TC6: Reserve"=w456:sgl, "TC7: Reserve"=w455:sgl)
      n218 = call "FGV FT-IR Diagnosewerte.vi"("Aktionen"=FGV_FT-IR_Diagnose_Aktionen."Lesen") -> ("Temperatur"=w466:dbl)  [unwired: 5 in, 5 out]
      n219 = Build Array(w466, w465, w464, w463, w462, w461, w457, w456, w455) -> (w460:dbl[])
      n220 = for {
        tunnel: w460 -> [w476] mode=indexing
        shift-right: [w471] -> w459
        shift-left: w458 -> [w474]
        n221 = Number To Fractional String(number=w476, precision (6)=i16 1 ("Genauigkeit (6)")) -> (F-format string=w472:string)  [unwired: 2 in]
        n222 = call <vilib>:"Space Constant.vi"() -> ("String"=w473:string)
        n223 = Concatenate Strings(w474, w473, w472) -> (w471:string)
      }
    }
    frame "AGTM" {
      # "Gaskühler Temp"
      # "#MEXA"
      n224 = call "Zustandsfehlerinformation.vi"("Aktionen"=Aktionen_Zustandsfehlerinformation."OK", "String"=w483) -> ("String"=w478:string)  [unwired: 9 in]
      n225 = call "FGV cRIO-Daten.vi"("Aktion"=enum16{"lesen", "schreiben"}."lesen") -> ("TC Eingänge"=w477:T41)  [unwired: 9 in, 9 out]
      n226 = Unbundle By Name(w477) -> ("TC0: Reserve"=w481:sgl)
      n227 = Build Array(w481) -> (w480:sgl[])
      n228 = for {
        tunnel: w480 -> [w490] mode=indexing
        shift-right: [w485] -> w479
        shift-left: w478 -> [w488]
        n229 = Number To Fractional String(number=w490, precision (6)=i16 1 ("Genauigkeit (6)")) -> (F-format string=w486:string)  [unwired: 2 in]
        n230 = call <vilib>:"Space Constant.vi"() -> ("String"=w487:string)
        n231 = Concatenate Strings(w488, w487, w486) -> (w485:string)
      }
    }
    frame "ADRU" {
      n232 = call "Zustandsfehlerinformation.vi"("Aktionen"=Aktionen_Zustandsfehlerinformation."OK", "String"=w506) -> ("String"=w500:string)  [unwired: 9 in]
      n233 = call "FGV cRIO-Daten.vi"("Aktion"=enum16{"lesen", "schreiben"}."lesen") -> ("Analog Input"=w504:T42)  [unwired: 9 in, 9 out]
      n234 = Unbundle By Name(w504) -> ("AI1: Druck Ausgang"=w496:sgl, "AI3: Druck FT-IR"=w494:sgl)
      n235 = call "FGV FT-IR Diagnosewerte.vi"("Aktionen"=FGV_FT-IR_Diagnose_Aktionen."Lesen") -> ("Druck"=w498:dbl)  [unwired: 5 in, 5 out]
      n236 = Number To Fractional String(number=w498, precision (6)=i16 3 ("Genauigkeit (6)")) -> (F-format string=w493:string)  [unwired: 2 in]
      n237 = Number To Fractional String(number=w496, precision (6)=i16 0 ("Genauigkeit (6)")) -> (F-format string=w491:string)  [unwired: 2 in]
      n238 = Number To Fractional String(number=w494, precision (6)=i16 1 ("Genauigkeit (6)")) -> (F-format string=w492:string)  [unwired: 2 in]
      n239 = Build Array(w493, w491, w492) -> (w502:string[])
      n240 = for {
        tunnel: w502 -> [w508] mode=indexing
        shift-right: [w509] -> w501
        shift-left: w500 -> [w511]
        n241 = call <vilib>:"Space Constant.vi"() -> ("String"=w510:string)
        n242 = Concatenate Strings(w511, w510, w508) -> (w509:string)
      }
    }
    frame "ADUF" {
      n243 = call "Zustandsfehlerinformation.vi"("Aktionen"=Aktionen_Zustandsfehlerinformation."OK", "String"=w520) -> ("String"=w516:string)  [unwired: 9 in]
      n244 = call "FGV cRIO-Daten.vi"("Aktion"=enum16{"lesen", "schreiben"}."lesen") -> ("Analog Input"=w519:T42)  [unwired: 9 in, 9 out]
      n245 = Unbundle By Name(w519) -> ("AI0: Durchfluss FT-IR"=w515:sgl)
      n246 = Number To Fractional String(number=w515, precision (6)=i16 1 ("Genauigkeit (6)")) -> (F-format string=w512:string)  [unwired: 2 in]
      n247 = call <vilib>:"Space Constant.vi"() -> ("String"=w513:string)
      n248 = Concatenate Strings(w516, w513, w512) -> (w517:string)
    }
    frame "AGID" {
      n249 = call "Zustandsfehlerinformation.vi"("Aktionen"=Aktionen_Zustandsfehlerinformation."OK", "String"=w527) -> ("String"=w524:string)  [unwired: 9 in]
      n250 = call "FGV System Konstanten.vi"("Aktionen"=Aktioen_FGV_System_Konstanten."lesen") -> ("LanguageList"=w523:string)  [unwired: 6 in, 4 out]
      n251 = call <vilib>:"Space Constant.vi"() -> ("String"=w526:string)
      n252 = Concatenate Strings(w524, w526, w523) -> (w522:string)
    }
    frame "AVER" {
      n253 = call "Zustandsfehlerinformation.vi"("Aktionen"=Aktionen_Zustandsfehlerinformation."OK", "String"=w535) -> ("String"=w532:string)  [unwired: 9 in]
      n254 = call "FGV System Konstanten.vi"("Aktionen"=Aktioen_FGV_System_Konstanten."lesen") -> ("Cluster out"=w530:T35)  [unwired: 6 in, 4 out]
      n255 = Unbundle By Name(w530) -> ("Software Version"=w529:string)
      n256 = call <vilib>:"Space Constant.vi"() -> ("String"=w534:string)
      n257 = Concatenate Strings(w532, w534, w529) -> (w531:string)
    }
    frame "ALEC" {
      n258 = call "Zustandsfehlerinformation.vi"("Aktionen"=Aktionen_Zustandsfehlerinformation."OK", "String"=w550) -> ("String"=w549:string)  [unwired: 9 in]
      n259 = call "Status Dichtheitstest.vi"("Aktionen"=Status_Dichtheitstest_Aktionen."lesen") -> ("Fehler"=w538:bool, "läuft?"=w542:bool, "Anstieg"=w547:sgl)  [unwired: 6 in, 2 out]
      n260 = Or(x=w542, y=w538) -> (x .or. y?=w541:bool)
      n261 = Number To Decimal String(number=w547) -> (decimal integer string=w546:string)  [unwired: 1 in]
      n262 = call <vilib>:"Space Constant.vi"() -> ("String"=w545:string)
      n263 = Concatenate Strings(w549, w545, w546) -> (w544:string)
      n264 = Select(t="error", s=w538, f="busy") -> (s? t:f=w537:string)
      n265 = case shown="True" w541 {
        tunnel: w544 -> [w552 w555]
        tunnel: [w552 w553] -> w543
        tunnel: w537 -> [_ w554]
        frame False {
        }
        frame True {
          n266 = call <vilib>:"Space Constant.vi"() -> ("String"=w556:string)
          n267 = Concatenate Strings(w555, w556, w554) -> (w553:string)
        }
      }
    }
    frame "ALES" {
      n268 = call "FGV Erweiterte Konfig.vi"("Aktion"=FGV_PID_Aktionen."Lesen") -> ("Sonstige"=w563:T43)  [unwired: 5 in, 5 out]
      n269 = call "Zustandsfehlerinformation.vi"("Aktionen"=Aktionen_Zustandsfehlerinformation."OK", "String"=w571) -> ("String"=w568:string)  [unwired: 9 in]
      n270 = Unbundle By Name(w563) -> ("Dichtheitstest Zeit"=w560:sgl, "Dichtheitstest Abfall"=w559:sgl, "Dichtheitstest Umfang"=w558:T45)
      n271 = Number To Fractional String(number=w560, precision (6)=i16 0 ("Genauigkeit (6)")) -> (F-format string=w557:string)  [unwired: 2 in]
      n272 = Number To Fractional String(number=w559, precision (6)=i16 0 ("Genauigkeit (6)")) -> (F-format string=w564:string)  [unwired: 2 in]
      n273 = Number To Fractional String(number=w558, precision (6)=i16 0 ("Genauigkeit (6)")) -> (F-format string=w565:string)  [unwired: 2 in]
      n274 = Build Array(w557, w564, w565) -> (w570:string[])
      n275 = for {
        tunnel: w570 -> [w573] mode=indexing
        shift-right: [w574] -> w569
        shift-left: w568 -> [w576]
        n276 = call <vilib>:"Space Constant.vi"() -> ("String"=w575:string)
        n277 = Concatenate Strings(w576, w575, w573) -> (w574:string)
      }
    }
    frame "ANOS" {
      n278 = call "Zustandsfehlerinformation.vi"("Aktionen"=Aktionen_Zustandsfehlerinformation."OK", "String"=w582) -> ("String"=w581:string)  [unwired: 9 in]
      n279 = call "FGV FT-IR Parameter.vi"("Aktion"=FGV_FT-IR_Aktionen."lesen") -> ("NoOfScan"=w577:u32)  [unwired: 11 in, 7 out]
      n280 = call <vilib>:"Space Constant.vi"() -> ("String"=w580:string)
      n281 = Number To Decimal String(number=w577) -> (decimal integer string=w579:string)  [unwired: 1 in]
      n282 = Concatenate Strings(w581, w580, w579) -> (w584:string)
    }
    frame "ALNB" {
      n283 = call "Zustandsfehlerinformation.vi"("Aktionen"=Aktionen_Zustandsfehlerinformation."OK", "String"=w591) -> ("String"=w590:string)  [unwired: 9 in]
      n284 = call "FGV Erweiterte Konfig.vi"("Aktion"=FGV_PID_Aktionen."Lesen") -> ("Sonstige"=w587:T43)  [unwired: 5 in, 5 out]
      n285 = Unbundle By Name(w587) -> ("Befüllung aktiv"=w585:T44)
      n286 = call <vilib>:"Space Constant.vi"() -> ("String"=w589:string)
      n287 = Number To Decimal String(number=w585) -> (decimal integer string=w588:string)  [unwired: 1 in]
      n288 = Concatenate Strings(w590, w589, w588) -> (w593:string)
    }
    frame "ADFT" {
      n289 = call "FGV Anlagengrenzwerte.vi"("Aktion"=FGV_Anlagengrenzwerte_Aktionen."Lesen") -> ("Anlagen-Grenzwerte Anzeige"=w597:T46)  [unwired: 1 in, 9 out]
      n290 = call "Zustandsfehlerinformation.vi"("Aktionen"=Aktionen_Zustandsfehlerinformation."OK", "String"=w601) -> ("String"=w600:string)  [unwired: 9 in]
      n291 = Unbundle By Name(w597) -> ("Durchfluss FT-IR:.Sollwert"=w596:sgl)
      n292 = call <vilib>:"Space Constant.vi"() -> ("String"=w599:string)
      n293 = Number To Fractional String(number=w596, precision (6)=i16 1 ("Genauigkeit (6)")) -> (F-format string=w594:string)  [unwired: 2 in]
      n294 = Concatenate Strings(w600, w599, w594) -> (w603:string)
    }
    frame "ABST" {
      n295 = call "Zustandsfehlerinformation.vi"("Aktionen"=Aktionen_Zustandsfehlerinformation."OK", "String"=w615) -> ("String"=w612:string)  [unwired: 9 in]
      n296 = call "FGV cRIO-Daten.vi"("Aktion"=enum16{"lesen", "schreiben"}."lesen") -> ("PID Stellwerte"=w604:i16[])  [unwired: 9 in, 9 out]
      n297 = Index Array(array=w604) -> (element #1=w605:i16, element #2=w606:i16)  [unwired: 2 in]
      n298 = Number To Fractional String(number=w605, precision (6)=i16 1 ("Genauigkeit (6)")) -> (F-format string=w609:string)  [unwired: 2 in]
      n299 = Number To Fractional String(number=w606, precision (6)=i16 1 ("Genauigkeit (6)")) -> (F-format string=w608:string)  [unwired: 2 in]
      n300 = Build Array(w609, w608) -> (w614:string[])
      n301 = for {
        tunnel: w614 -> [w617] mode=indexing
        shift-right: [w618] -> w613
        shift-left: w612 -> [w620]
        n302 = call <vilib>:"Space Constant.vi"() -> ("String"=w619:string)
        n303 = Concatenate Strings(w620, w619, w617) -> (w618:string)
      }
    }
    frame "SECO" {
      n304 = call "Setze Zustand.vi"("AK Befehl"=w623, "Zustand"=Zustaende."Eco") -> ("Antwort String"=w622:string)  [unwired: 8 in, 1 out]
    }
    frame "SPAU" {
      n305 = call "Setze Zustand.vi"("AK Befehl"=w626, "Zustand"=Zustaende."Pause") -> ("Antwort String"=w625:string)  [unwired: 8 in, 1 out]
    }
    frame "STBY" {
      n306 = call "Setze Zustand.vi"("AK Befehl"=w629, "Zustand"=Zustaende."Standby") -> ("Antwort String"=w628:string)  [unwired: 8 in, 1 out]
    }
    frame "SMGA" {
      n307 = call "Setze Zustand.vi"("AK Befehl"=w632, "Zustand"=Zustaende."Messen") -> ("Antwort String"=w631:string)  [unwired: 8 in, 1 out]
    }
    frame "SSPL" {
      n308 = Index Array(array=w634, index=2 ("Index")) -> (element=w638:string)
      n309 = Decimal String To Number(string=w638) -> (number=w637:i32)  [unwired: 2 in, 1 out]
      n310 = Divide(x=w637, y=10) -> (x/y=w635:dbl)
      n311 = To Single Precision Float(number=w635) -> (single precision float=w633:sgl)
      n312 = call "Setze Zustand.vi"("Zeit"=w633, "AK Befehl"=w642, "Zustand"=Zustaende."Spülen Leitung") -> ("Antwort String"=w641:string)  [unwired: 7 in, 1 out]
    }
    frame "SRUC" {
      n313 = Index Array(array=w644, index=2 ("Index")) -> (element=w648:string)
      n314 = Decimal String To Number(string=w648) -> (number=w647:i32)  [unwired: 2 in, 1 out]
      n315 = Divide(x=w647, y=10) -> (x/y=w645:dbl)
      n316 = To Single Precision Float(number=w645) -> (single precision float=w643:sgl)
      n317 = call "Setze Zustand.vi"("Zeit"=w643, "AK Befehl"=w652, "Zustand"=Zustaende."Spülen Filter") -> ("Antwort String"=w651:string)  [unwired: 7 in, 1 out]
    }
    frame "SSPR" {
      n318 = call "Setze Zustand.vi"("Befehl nicht vorhanden!"=TRUE, "AK Befehl"=w656, "Zustand"=Zustaende."Standby") -> ("Antwort String"=w655:string)  [unwired: 7 in, 1 out]
    }
    frame "SNGA" {
      n319 = Index Array(array=w664, index=2 ("Index")) -> (element=w662:string)
      n320 = Decimal String To Number(string=w662) -> (number=w661:i32)  [unwired: 2 in, 1 out]
      n321 = Divide(x=w661, y=10) -> (x/y=w659:dbl)
      n322 = To Single Precision Float(number=w659) -> (single precision float=w657:sgl)
      n323 = call "Setze Zustand.vi"("Zeit"=w657, "AK Befehl"=w666, "Zustand"=Zustaende."0-Gas") -> ("Antwort String"=w665:string)  [unwired: 7 in, 1 out]
    }
    frame "SNGF" {
      n324 = call "Setze Zustand.vi"("Befehl nicht vorhanden!"=TRUE, "AK Befehl"=w670, "Zustand"=Zustaende."Standby") -> ("Antwort String"=w669:string)  [unwired: 7 in, 1 out]
    }
    frame "SMAN" {
      n325 = call "FGV-Funktionstasten.vi"("Aktion"=Funktionstasten-Aktion."Lesen") -> ("Betriebsart"=w676:T22)  [unwired: 7 in, 7 out]
      n326 = Equal?(x=w676, y=Betriebsart."Remote" ("Betriebsart")) -> (x = y?=w673:bool)
      n327 = case shown="True" w673 {
        tunnel: w672 -> [w679 w682]
        tunnel: [w677 w681] -> w671
        frame False {
          n328 = call "Zustandsfehlerinformation.vi"("Aktionen"=Aktionen_Zustandsfehlerinformation."Offline", "String"=w679) -> ("String"=w677:string)  [unwired: 9 in]
        }
        frame True {
          n329 = call "Zustandsfehlerinformation.vi"("Aktionen"=Aktionen_Zustandsfehlerinformation."OK", "String"=w682) -> ("String"=w681:string)  [unwired: 9 in]
          n330 = call "FGV-Funktionstasten.vi"("Aktion"=Funktionstasten-Aktion."Manuell") -> ()  [unwired: 7 in, 8 out]
        }
      }
    }
    frame "SREM" {
      n331 = call "Zustandsfehlerinformation.vi"("Aktionen"=Aktionen_Zustandsfehlerinformation."OK", "String"=w685) -> ("String"=w684:string)  [unwired: 9 in]
      n332 = call "FGV-Funktionstasten.vi"("Aktion"=Funktionstasten-Aktion."Remote") -> ()  [unwired: 7 in, 8 out]
    }
    frame "SEMB" {
      n333 = call "FGV-Funktionstasten.vi"("Aktion"=Funktionstasten-Aktion."Lesen") -> ("Betriebsart"=w694:T22)  [unwired: 7 in, 7 out]
      n334 = Equal?(x=w694, y=Betriebsart."Remote" ("Betriebsart")) -> ()  [unwired: 1 out]
      n335 = case shown="True" TRUE {
        tunnel: w691 -> [w696 w704]
        tunnel: [w695 w703] -> w690
        tunnel: w689 -> [_ w702]
        frame False {
          n336 = call "Zustandsfehlerinformation.vi"("Aktionen"=Aktionen_Zustandsfehlerinformation."Offline", "String"=w696) -> ("String"=w695:string)  [unwired: 9 in]
        }
        frame True {
          # "Messbereich FID via AK"
          # "#MEXA"
          n337 = Index Array(array=w702, index=2 ("Index")) -> (element=w700:string)
          n338 = call "Zustandsfehlerinformation.vi"("Aktionen"=Aktionen_Zustandsfehlerinformation."OK", "String"=w704) -> ("String"=w703:string)  [unwired: 9 in]
          n339 = Decimal String To Number(string=w700, offset=1 ("Offset (0)")) -> (number=w698:i32)  [unwired: 1 in, 1 out]
          n340 = stacked-sequence {
            tunnel: w698 -> [w706 _]
            frame #0 {
              n341 = call "FGV Analysator Definition.vi"("Aktionen"=FGV_Analysator_Definition_Aktionen."MB setzen", "Messbereich"=w706, "Komponente"=1) -> ()  [unwired: 4 in, 5 out]
            }
            frame #1 {
              # "Namen ändern"
              n342 = call "Namen in der Gasliste aendern.vi"() -> ()  [unwired: 12 in]
            }
          }
        }
      }
    }
    frame "SEGA" {
      n343 = call "FGV-Funktionstasten.vi"("Aktion"=Funktionstasten-Aktion."Lesen") -> ("Betriebsart"=w713:T22)  [unwired: 7 in, 7 out]
      n344 = Equal?(x=w713, y=Betriebsart."Remote" ("Betriebsart")) -> (x = y?=w714:bool)
      n345 = case shown="True" w714 {
        tunnel: w710 -> [w716 w721]
        tunnel: [w715 w720] -> w709
        frame False {
          n346 = call "Zustandsfehlerinformation.vi"("Aktionen"=Aktionen_Zustandsfehlerinformation."Offline", "String"=w716) -> ("String"=w715:string)  [unwired: 9 in]
        }
        frame True {
          n347 = call "Gespeicherte Werte.vi"("Aktionen"=Aktionen_Gespeicherte_Werte."lesen") -> ("Diverse Werte"=w722:T37)  [unwired: 6 in, 4 out]
          n348 = Unbundle By Name(w722) -> ("Kalibriergaseingang"=w718:i16)
          n349 = case shown="0, Standard" w718 {
            tunnel: [Zustaende."Standby" ("Zustand") Zustaende."Cal-Gas" ("Zustand")] -> w719
            frame 0, Default {
            }
            frame 1..3 {
            }
          }
          n350 = call "Setze Zustand.vi"("AK Befehl"=w721, "Zustand"=w719) -> ("Antwort String"=w720:string)  [unwired: 8 in, 1 out]
        }
      }
    }
    frame "SATK" {
      n351 = call "Setze Zustand.vi"("AK Befehl"=w727, "Zustand"=Zustaende."Kalibrieren") -> ("Antwort String"=w726:string)  [unwired: 8 in, 1 out]
    }
    frame "SENT" {
      n352 = call "FGV-Funktionstasten.vi"("Aktion"=Funktionstasten-Aktion."Lesen") -> ("Betriebsart"=w735:T22)  [unwired: 7 in, 7 out]
      n353 = Equal?(x=w735, y=Betriebsart."Remote" ("Betriebsart")) -> (x = y?=w729:bool)
      n354 = case shown="True" w729 {
        tunnel: w732 -> [w737 w746]
        tunnel: [w736 w745] -> w731
        tunnel: w730 -> [_ w744]
        frame False {
          n355 = call "Zustandsfehlerinformation.vi"("Aktionen"=Aktionen_Zustandsfehlerinformation."Offline", "String"=w737) -> ("String"=w736:string)  [unwired: 9 in]
        }
        frame True {
          n356 = call "Zustandsfehlerinformation.vi"("Aktionen"=Aktionen_Zustandsfehlerinformation."OK", "String"=w746) -> ("String"=w745:string)  [unwired: 9 in]
          n357 = for {
            tunnel: w744 -> [w751] mode=indexing
            shift-right: [w750] -> w743
            shift-left: "" -> [w749]
            n358 = call <vilib>:"Space Constant.vi"() -> ("String"=w748:string)
            n359 = Concatenate Strings(w749, w748, w751) -> (w750:string)
          }
          n360 = String Subset(string=w743, offset (0)=1 ("Offset (0)")) -> (substring=w740:string)  [unwired: 1 in]
          n361 = call "Amium Kommandos verwalten.vi"("Aktionen"=Amium_Kommandos_verwalten_Aktionen."setzen Pos1", "neues Kommando"=w740) -> ()  [unwired: 7 in, 3 out]
        }
      }
    }
    frame "STRG" {
      n362 = call "FGV-Funktionstasten.vi"("Aktion"=Funktionstasten-Aktion."Lesen") -> ("Betriebsart"=w757:T22)  [unwired: 7 in, 7 out]
      n363 = Equal?(x=w757, y=Betriebsart."Remote" ("Betriebsart")) -> (x = y?=w758:bool)
      n364 = case shown="True" w758 {
        tunnel: w754 -> [w760 w767]
        tunnel: [w759 w766] -> w753
        tunnel: w752 -> [_ w765]
        frame False {
          n365 = call "Zustandsfehlerinformation.vi"("Aktionen"=Aktionen_Zustandsfehlerinformation."Offline", "String"=w760) -> ("String"=w759:string)  [unwired: 9 in]
        }
        frame True {
          n366 = Index Array(array=w765, index=2 ("Index")) -> (element=w763:string)
          n367 = Empty String/Path?(string/path=w763) -> (empty?=w762:bool)
          n368 = case shown="False" w762 {
            tunnel: w767 -> [w774 w787]
            tunnel: [w773 w786] -> w766
            tunnel: w763 -> [w772 _]
            frame False {
              n369 = Decimal String To Number(string=w772) -> (number=w769:i32)  [unwired: 2 in, 1 out]
              n370 = In Range and Coerce(upper limit=2 ("Obergrenze"), x=w769, lower limit=0 ("Untergrenze")) -> (In Range?=w768:bool)  [unwired: 1 out]
              n371 = case shown="True" w768 {
                tunnel: w774 -> [w776 w784]
                tunnel: [w775 w783] -> w773
                tunnel: w769 -> [_ w778]
                frame False {
                  n372 = call "Zustandsfehlerinformation.vi"("Aktionen"=Aktionen_Zustandsfehlerinformation."Datenfehler", "String"=w776) -> ("String"=w775:string)  [unwired: 9 in]
                }
                frame True {
                  # "Wenn informationen da sind, dann übergeben!"
                  n373 = call "FGV Trigger.vi"("Aktion"=Aktionen_Trigger."lesen") -> ("Triggerereignis neu"=w780:T48)  [unwired: 7 in, 3 out]
                  n374 = Bundle By Name(cluster=w780, "Trigger verwenden"=w778) -> (w779:T48)
                  n375 = call "Zustandsfehlerinformation.vi"("Aktionen"=Aktionen_Zustandsfehlerinformation."OK", "String"=w784) -> ("String"=w783:string)  [unwired: 9 in]
                  n376 = call "FGV Trigger.vi"("Aktion"=Aktionen_Trigger."ALLE schreiben", "Triggerereignis"=w779) -> ()  [unwired: 6 in, 4 out]
                }
              }
            }
            frame True {
              # "Wenn nur STRG dann Trigger setzen!!!"
              n377 = call "FGV Trigger.vi"("Aktion"=Aktionen_Trigger."Trigger prüfen", "Trigger setzen"=TRUE) -> ()  [unwired: 6 in, 4 out]
              n378 = call "Zustandsfehlerinformation.vi"("Aktionen"=Aktionen_Zustandsfehlerinformation."OK", "String"=w787) -> ("String"=w786:string)  [unwired: 9 in]
            }
          }
        }
      }
    }
    frame "SLEC" {
      n379 = call "FGV-Funktionstasten.vi"("Aktion"=Funktionstasten-Aktion."Lesen") -> ("ausgewählte Funktion"=w791:T12, "Betriebsart"=w796:T22)  [unwired: 7 in, 6 out]
      n380 = Equal?(x=w796, y=Betriebsart."Remote" ("Betriebsart")) -> (x = y?=w797:bool)
      n381 = case shown="True" w797 {
        tunnel: w793 -> [w799 w805]
        tunnel: [w798 w804] -> w792
        tunnel: w791 -> [_ w803]
        frame False {
          n382 = call "Zustandsfehlerinformation.vi"("Aktionen"=Aktionen_Zustandsfehlerinformation."Offline", "String"=w799) -> ("String"=w798:string)  [unwired: 9 in]
        }
        frame True {
          n383 = Equal?(x=w803, y=Zustaende."Standby") -> (x = y?=w801:bool)
          n384 = case shown="True" w801 {
            tunnel: w805 -> [w808 w810]
            tunnel: [w807 w809] -> w804
            frame False {
              n385 = call "Zustandsfehlerinformation.vi"("Aktionen"=Aktionen_Zustandsfehlerinformation."Datenfehler", "String"=w808) -> ("String"=w807:string)  [unwired: 9 in]
            }
            frame True {
              n386 = flat-sequence {
                frame #0 {
                  n387 = call "FGV Erweiterte Konfig.vi"("Aktion"=FGV_PID_Aktionen."Dichtheitstest", "Dichtheitstest?"=TRUE) -> ()  [unwired: 5 in, 5 out]
                }
                frame #1 {
                  n388 = vi-ref "Erweiterte Konfig.lvlib:Dichtheitstest.vi"() -> (w814:refnum<vi>)
                  n389 = call "VI Pop Up.vi"("VI Referenz"=w814) -> ()  [unwired: 10 in, 1 out]
                }
              }
              n390 = call "Zustandsfehlerinformation.vi"("Aktionen"=Aktionen_Zustandsfehlerinformation."OK", "String"=w810) -> ("String"=w809:string)  [unwired: 9 in]
            }
          }
        }
      }
    }
    frame "SLES" {
      n391 = call "FGV-Funktionstasten.vi"("Aktion"=Funktionstasten-Aktion."Lesen") -> ("Betriebsart"=w820:T22)  [unwired: 7 in, 7 out]
      n392 = Equal?(x=w820, y=Betriebsart."Remote" ("Betriebsart")) -> (x = y?=w821:bool)
      n393 = case shown="True" w821 {
        tunnel: w817 -> [w823 w856]
        tunnel: [w822 w855] -> w816
        tunnel: w815 -> [_ w854]
        frame False {
          n394 = call "Zustandsfehlerinformation.vi"("Aktionen"=Aktionen_Zustandsfehlerinformation."Offline", "String"=w823) -> ("String"=w822:string)  [unwired: 9 in]
        }
        frame True {
          n395 = Index Array(array=w854, index #1=2 ("Index"), index #2=3 ("Index"), index #3=4 ("Index")) -> (element #1=w828:string, element #2=w829:string, element #3=w830:string)
          n396 = Empty String/Path?(string/path=w828) -> (empty?=w833:bool)
          n397 = Empty String/Path?(string/path=w829) -> (empty?=w832:bool)
          n398 = Empty String/Path?(string/path=w830) -> (empty?=w831:bool)
          n399 = Decimal String To Number(string=w828) -> (number=w850:i32)  [unwired: 2 in, 1 out]
          n400 = Decimal String To Number(string=w829) -> (number=w846:i32)  [unwired: 2 in, 1 out]
          n401 = Decimal String To Number(string=w830) -> (number=w841:i32)  [unwired: 2 in, 1 out]
          n402 = Not(x=w833) -> (.not. x?=w827:bool)
          n403 = Not(x=w832) -> (.not. x?=w826:bool)
          n404 = Not(x=w831) -> (.not. x?=w825:bool)
          n405 = In Range and Coerce(upper limit=101 ("Obergrenze"), x=w850, lower limit=1 ("Untergrenze")) -> (coerced(x)=w836:i32, In Range?=w838:bool)
          n406 = In Range and Coerce(upper limit=101 ("Obergrenze"), x=w846, lower limit=1 ("Untergrenze")) -> (coerced(x)=w835:i32, In Range?=w839:bool)
          n407 = In Range and Coerce(upper limit=3 ("Obergrenze"), x=w841, lower limit=0 ("Untergrenze")) -> (coerced(x)=w834:i32, In Range?=w840:bool)
          n408 = Compound Arithmetic op=AND(w838, w839, w840, w827, w826, w825) -> (w837:bool)
          n409 = case shown="True" w837 {
            tunnel: [Aktionen_Zustandsfehlerinformation."Datenfehler" ("Aktionen") Aktionen_Zustandsfehlerinformation."OK" ("Aktionen")] -> w849
            tunnel: w836 -> [_ w860]
            tunnel: w835 -> [_ w859]
            tunnel: w834 -> [_ w858]
            frame False {
            }
            frame True {
              n410 = call "FGV Erweiterte Konfig.vi"("Aktion"=FGV_PID_Aktionen."Lesen") -> ("Sonstige"=w863:T43)  [unwired: 5 in, 5 out]
              n411 = Bundle By Name(cluster=w863, "Dichtheitstest Zeit"=w860, "Dichtheitstest Abfall"=w859, "Dichtheitstest Umfang"=w858) -> (w864:T43)
              n412 = call "FGV Erweiterte Konfig.vi"("Aktion"=FGV_PID_Aktionen."Schreiben Sonstige", "Sonstige"=w864) -> ()  [unwired: 4 in, 6 out]
            }
          }
          n413 = call "Zustandsfehlerinformation.vi"("Aktionen"=w849, "String"=w856) -> ("String"=w855:string)  [unwired: 9 in]
        }
      }
    }
    frame "SLNB" {
      n414 = call "FGV-Funktionstasten.vi"("Aktion"=Funktionstasten-Aktion."Lesen") -> ("Betriebsart"=w871:T22)  [unwired: 7 in, 7 out]
      n415 = Equal?(x=w871, y=Betriebsart."Remote" ("Betriebsart")) -> (x = y?=w872:bool)
      n416 = case shown="True" w872 {
        tunnel: w868 -> [w874 w889]
        tunnel: [w873 w888] -> w867
        tunnel: w866 -> [_ w887]
        frame False {
          n417 = call "Zustandsfehlerinformation.vi"("Aktionen"=Aktionen_Zustandsfehlerinformation."Offline", "String"=w874) -> ("String"=w873:string)  [unwired: 9 in]
        }
        frame True {
          # "0 oder 1"
          n418 = Index Array(array=w887, index=2 ("Index")) -> (element=w878:string)
          n419 = Decimal String To Number(string=w878) -> (number=w883:i32)  [unwired: 2 in, 1 out]
          n420 = Empty String/Path?(string/path=w878) -> (empty?=w877:bool)
          n421 = In Range and Coerce(upper limit=2 ("Obergrenze"), x=w883, lower limit=0 ("Untergrenze")) -> (coerced(x)=w879:i32, In Range?=w881:bool)
          n422 = Not(x=w877) -> (.not. x?=w876:bool)
          n423 = And(x=w881, y=w876) -> (x .and. y?=w880:bool)
          n424 = case shown="True" w880 {
            tunnel: [Aktionen_Zustandsfehlerinformation."Datenfehler" ("Aktionen") Aktionen_Zustandsfehlerinformation."OK" ("Aktionen")] -> w882
            tunnel: w879 -> [_ w891]
            frame False {
            }
            frame True {
              n425 = call "FGV Erweiterte Konfig.vi"("Aktion"=FGV_PID_Aktionen."Lesen") -> ("Sonstige"=w894:T43)  [unwired: 5 in, 5 out]
              n426 = Bundle By Name(cluster=w894, "Befüllung aktiv"=w891) -> (w895:T43)
              n427 = call "FGV Erweiterte Konfig.vi"("Aktion"=FGV_PID_Aktionen."Schreiben Sonstige", "Sonstige"=w895) -> ()  [unwired: 4 in, 6 out]
            }
          }
          n428 = call "Zustandsfehlerinformation.vi"("Aktionen"=w882, "String"=w889) -> ("String"=w888:string)  [unwired: 9 in]
        }
      }
    }
    frame "SNOS" {
      n429 = call "FGV-Funktionstasten.vi"("Aktion"=Funktionstasten-Aktion."Lesen") -> ("Betriebsart"=w902:T22)  [unwired: 7 in, 7 out]
      n430 = Equal?(x=w902, y=Betriebsart."Remote" ("Betriebsart")) -> (x = y?=w903:bool)
      n431 = case shown="True" w903 {
        tunnel: w899 -> [w905 w917]
        tunnel: [w904 w916] -> w898
        tunnel: w897 -> [_ w915]
        frame False {
          n432 = call "Zustandsfehlerinformation.vi"("Aktionen"=Aktionen_Zustandsfehlerinformation."Offline", "String"=w905) -> ("String"=w904:string)  [unwired: 9 in]
        }
        frame True {
          n433 = Index Array(array=w915, index=2 ("Index")) -> (element=w913:string)
          n434 = Decimal String To Number(string=w913) -> (number=w910:i32)  [unwired: 2 in, 1 out]
          n435 = In Range and Coerce(upper limit=101 ("Obergrenze"), x=w910, lower limit=1 ("Untergrenze")) -> (coerced(x)=w909:i32, In Range?=w908:bool)
          n436 = case shown="True" w908 {
            tunnel: w909 -> [_ w919]
            tunnel: [Aktionen_Zustandsfehlerinformation."Datenfehler" ("Aktionen") Aktionen_Zustandsfehlerinformation."OK" ("Aktionen")] -> w907
            frame False {
            }
            frame True {
              n437 = flat-sequence {
                tunnel: w919 -> [w921]
                frame #0 {
                  n438 = call "FGV FT-IR Parameter.vi"("NoOfScan neu"=w921, "Aktion"=FGV_FT-IR_Aktionen."NOS setzen") -> ("NoOfScan"=w922:u32)  [unwired: 10 in, 7 out]
                  n439 = call "TOOLweb SET ftirScans.vi"("ftirScans"=w922) -> ()  [unwired: 2 in, 5 out]
                }
                frame #1 {
                  n440 = call "Queue LogFile.vi"() -> ("error out"=w927:errorcluster, "Queue (Ausgang)"=w926:refnum<queue>)  [unwired: 6 in]
                  n441 = call "FGV Messdaten.vi"("Aktionen"=Aktionen_FGV_Messdaten."löschen") -> ()  [unwired: 6 in, 9 out]
                  n442 = Flush Queue(queue=w926, error in (no error)=w927) -> (error out=w924:errorcluster)  [unwired: 2 out]
                  n443 = call <vilib>:"Clear Errors.vi"("error in (no error)"=w924) -> ()  [unwired: 5 in, 2 out]
                }
              }
            }
          }
          n444 = call "Zustandsfehlerinformation.vi"("Aktionen"=w907, "String"=w917) -> ("String"=w916:string)  [unwired: 9 in]
        }
      }
    }
  }
  "String für schreiben" <- w5
